vi "Check Path Length.vi"(8 "y":i32) -> (2 "Array":cluster{string, i32}[](array[cluster])=[{"", 141}, {"", 140}, {"", 145}, {"", 139}, {"", 129}, {"", 148}, {"", 114}, {"", 129}, {"", 127}, {"", 158}, {"", 146}, {"", 158}, {"", 147}, {"", 146}, {"", 152}, {"", 148}, {"", 155}, {"", 135}, {"", 149}, {"", 136}, {"", 152}, {"", 149}, {"", 154}, {"", 162}, {"", 163}, {"", 147}, {"", 177}, {"", 166}, {"", 149}, {"", 134}, {"", 134}, {"", 157}, {"", 167}, {"", 153}, {"", 153}, {"", 140}, {"", 159}, {"", 160}, {"", 163}, {"", 168}, {"", 167}, {"", 147}, {"", 161}, {"", 135}, {"", 147}, {"", 160}, {"", 161}, {"", 149}, {"", 156}, {"", 132}, {"", 128}, {"", 151}, {"", 154}, {"", 156}, {"", 160}, {"", 148}, {"", 143}, {"", 147}, {"", 143}, {"", 141}, {"", 143}, {"", 140}, {"", 170}, {"", 147}, {"", 147}, {"", 135}, {"", 134}, {"", 129}, {"", 179}, {"", 180}, {"", 166}, {"", 161}, {"", 175}, {"", 178}, {"", 186}, {"", 160}, {"", 160}, {"", 148}, {"", 152}, {"", 146}, {"", 152}, {"", 150}, {"", 150}, {"", 151}, {"", 151}, {"", 151}, {"", 141}, {"", 166}, {"", 154}, {"", 154}, {"", 155}, {"", 156}, {"", 167}, {"", 155}, {"", 171}, {"", 169}, {"", 158}, {"", 143}, {"", 160}, {"", 141}, {"", 156}, {"", 143}, {"", 151}, {"", 158}, {"", 159}, {"", 147}, {"", 154}, {"", 152}, {"", 150}, {"", 153}, {"", 161}, {"", 151}, {"", 144}, {"", 149}, {"", 145}, {"", 144}, {"", 150}, {"", 158}, {"", 159}, {"", 157}, {"", 154}, {"", 150}, {"", 154}, {"", 142}, {"", 152}, {"", 146}, {"", 152}, {"", 151}, {"", 144}, {"", 148}, {"", 136}, {"", 150}, {"", 154}, {"", 149}, {"", 129}, {"", 162}, {"", 163}, {"", 164}, {"", 160}, {"", 163}, {"", 152}, {"", 162}, {"", 172}, {"", 149}, {"", 151}, {"", 162}, {"", 153}, {"", 163}, {"", 162}, {"", 158}, {"", 170}, {"", 165}, {"", 163}, {"", 163}, {"", 173}, {"", 155}, {"", 174}, {"", 173}, {"", 169}, {"", 166}, {"", 159}, {"", 160}, {"", 153}, {"", 143}, {"", 144}, {"", 138}, {"", 139}, {"", 136}, {"", 147}, {"", 148}, {"", 144}, {"", 151}, {"", 154}, {"", 131}, {"", 128}, {"", 170}, {"", 146}, {"", 140}, {"", 157}, {"", 151}, {"", 152}, {"", 152}, {"", 151}, {"", 162}, {"", 145}, {"", 144}, {"", 145}, {"", 150}, {"", 162}, {"", 170}, {"", 135}, {"", 131}, {"", 131}, {"", 159}, {"", 142}, {"", 157}, {"", 157}, {"", 147}, {"", 149}, {"", 160}, {"", 145}, {"", 150}, {"", 147}, {"", 164}, {"", 153}, {"", 175}, {"", 158}, {"", 146}, {"", 142}, {"", 144}, {"", 154}, {"", 151}, {"", 151}, {"", 152}, {"", 147}, {"", 144}, {"", 146}, {"", 146}, {"", 152}, {"", 143}, {"", 146}, {"", 142}, {"", 158}, {"", 149}, {"", 144}, {"", 151}, {"", 137}, {"", 152}, {"", 160}, {"", 142}, {"", 164}, {"", 145}, {"", 141}, {"", 144}, {"", 138}, {"", 139}, {"", 149}, {"", 161}, {"", 138}, {"", 166}, {"", 132}, {"", 140}, {"", 136}, {"", 139}, {"", 140}, {"", 132}, {"", 137}, {"", 146}, {"", 143}, {"", 144}, {"", 148}, {"", 141}, {"", 149}, {"", 150}, {"", 179}, {"", 162}, {"", 175}, {"", 168}, {"", 169}, {"", 155}, {"", 150}, {"", 149}, {"", 155}, {"", 152}, {"", 180}, {"", 163}, {"", 163}, {"", 160}, {"", 160}, {"", 157}, {"", 158}, {"", 163}, {"", 165}, {"", 157}, {"", 165}, {"", 161}, {"", 155}, {"", 159}, {"", 160}, {"", 147}, {"", 166}, {"", 151}, {"", 150}, {"", 162}, {"", 158}, {"", 171}, {"", 155}, {"", 167}, {"", 169}, {"", 167}, {"", 171}, {"", 167}, {"", 171}, {"", 169}, {"", 173}, {"", 175}, {"", 162}, {"", 174}, {"", 172}, {"", 176}, {"", 173}, {"", 177}, {"", 175}, {"", 179}, {"", 175}, {"", 163}, {"", 149}, {"", 160}, {"", 151}, {"", 153}, {"", 149}, {"", 149}, {"", 150}, {"", 146}, {"", 155}, {"", 153}, {"", 156}, {"", 142}, {"", 141}, {"", 143}, {"", 143}, {"", 147}, {"", 141}, {"", 149}, {"", 149}, {"", 153}, {"", 157}, {"", 164}, {"", 162}, {"", 162}, {"", 146}, {"", 151}, {"", 153}, {"", 137}, {"", 141}, {"", 145}, {"", 156}, {"", 151}, {"", 147}, {"", 146}, {"", 145}, {"", 149}, {"", 145}, {"", 142}, {"", 145}, {"", 149}, {"", 150}, {"", 144}, {"", 148}, {"", 160}, {"", 148}, {"", 176}, {"", 144}, {"", 146}, {"", 153}, {"", 136}, {"", 136}, {"", 147}, {"", 163}, {"", 175}, {"", 178}, {"", 189}, {"", 177}, {"", 144}, {"", 157}, {"", 160}, {"", 171}, {"", 159}, {"", 179}, {"", 170}, {"", 176}, {"", 121}, {"", 178}, {"", 178}, {"", 179}, {"", 181}, {"", 182}, {"", 178}, {"", 177}, {"", 156}, {"", 183}, {"", 183}, {"", 181}, {"", 175}, {"", 165}, {"", 182}, {"", 191}, {"", 185}, {"", 158}, {"", 150}, {"", 181}, {"", 154}, {"", 177}, {"", 170}, {"", 208}, {"", 179}, {"", 191}, {"", 200}, {"", 183}, {"", 186}, {"", 198}, {"", 170}, {"", 183}, {"", 181}, {"", 181}, {"", 183}, {"", 198}, {"", 186}, {"", 176}, {"", 174}, {"", 181}, {"", 180}, {"", 182}, {"", 181}, {"", 196}, {"", 194}, {"", 192}, {"", 189}, {"", 195}, {"", 183}, {"", 147}, {"", 146}, {"", 142}, {"", 141}, {"", 128}, {"", 173}, {"", 168}, {"", 170}, {"", 154}, {"", 149}, {"", 171}, {"", 161}, {"", 158}, {"", 184}, {"", 162}, {"", 134}, {"", 178}, {"", 171}, {"", 185}, {"", 171}, {"", 167}, {"", 167}, {"", 169}, {"", 140}, {"", 169}, {"", 157}, {"", 168}, {"", 182}, {"", 186}, {"", 184}, {"", 148}, {"", 173}, {"", 141}, {"", 130}, {"", 154}, {"", 138}, {"", 131}, {"", 140}, {"", 132}, {"", 160}, {"", 150}, {"", 150}, {"", 154}, {"", 149}, {"", 175}, {"", 150}, {"", 152}, {"", 149}, {"", 152}, {"", 147}, {"", 149}, {"", 151}, {"", 154}, {"", 160}, {"", 144}, {"", 166}, {"", 148}, {"", 155}, {"", 151}, {"", 155}, {"", 151}, {"", 143}, {"", 159}, {"", 135}, {"", 159}, {"", 175}, {"", 139}, {"", 159}, {"", 160}, {"", 153}, {"", 147}, {"", 148}, {"", 140}, {"", 144}, {"", 140}, {"", 147}, {"", 146}, {"", 139}, {"", 149}, {"", 163}, {"", 162}, {"", 165}, {"", 165}, {"", 154}, {"", 155}, {"", 137}, {"", 158}, {"", 147}, {"", 146}, {"", 151}, {"", 148}, {"", 158}, {"", 159}, {"", 155}, {"", 154}, {"", 125}, {"", 138}, {"", 131}, {"", 144}, {"", 139}, {"", 133}, {"", 140}, {"", 137}, {"", 145}, {"", 131}, {"", 146}, {"", 138}, {"", 122}, {"", 143}, {"", 138}, {"", 140}, {"", 146}, {"", 147}, {"", 140}, {"", 136}, {"", 140}, {"", 139}, {"", 134}, {"", 138}, {"", 122}, {"", 147}, {"", 155}, {"", 159}, {"", 142}, {"", 147}, {"", 145}, {"", 140}, {"", 150}, {"", 142}, {"", 150}, {"", 147}, {"", 167}, {"", 163}, {"", 165}], 3 "Waveform Graph":i32[](graph)=[141, 140, 145, 139, 129, 148, 114, 129, 127, 158, 146, 158, 147, 146, 152, 148, 155, 135, 149, 136, 152, 149, 154, 162, 163, 147, 177, 166, 149, 134, 134, 157, 167, 153, 153, 140, 159, 160, 163, 168, 167, 147, 161, 135, 147, 160, 161, 149, 156, 132, 128, 151, 154, 156, 160, 148, 143, 147, 143, 141, 143, 140, 170, 147, 147, 135, 134, 129, 179, 180, 166, 161, 175, 178, 186, 160, 160, 148, 152, 146, 152, 150, 150, 151, 151, 151, 141, 166, 154, 154, 155, 156, 167, 155, 171, 169, 158, 143, 160, 141, 156, 143, 151, 158, 159, 147, 154, 152, 150, 153, 161, 151, 144, 149, 145, 144, 150, 158, 159, 157, 154, 150, 154, 142, 152, 146, 152, 151, 144, 148, 136, 150, 154, 149, 129, 162, 163, 164, 160, 163, 152, 162, 172, 149, 151, 162, 153, 163, 162, 158, 170, 165, 163, 163, 173, 155, 174, 173, 169, 166, 159, 160, 153, 143, 144, 138, 139, 136, 147, 148, 144, 151, 154, 131, 128, 170, 146, 140, 157, 151, 152, 152, 151, 162, 145, 144, 145, 150, 162, 170, 135, 131, 131, 159, 142, 157, 157, 147, 149, 160, 145, 150, 147, 164, 153, 175, 158, 146, 142, 144, 154, 151, 151, 152, 147, 144, 146, 146, 152, 143, 146, 142, 158, 149, 144, 151, 137, 152, 160, 142, 164, 145, 141, 144, 138, 139, 149, 161, 138, 166, 132, 140, 136, 139, 140, 132, 137, 146, 143, 144, 148, 141, 149, 150, 179, 162, 175, 168, 169, 155, 150, 149, 155, 152, 180, 163, 163, 160, 160, 157, 158, 163, 165, 157, 165, 161, 155, 159, 160, 147, 166, 151, 150, 162, 158, 171, 155, 167, 169, 167, 171, 167, 171, 169, 173, 175, 162, 174, 172, 176, 173, 177, 175, 179, 175, 163, 149, 160, 151, 153, 149, 149, 150, 146, 155, 153, 156, 142, 141, 143, 143, 147, 141, 149, 149, 153, 157, 164, 162, 162, 146, 151, 153, 137, 141, 145, 156, 151, 147, 146, 145, 149, 145, 142, 145, 149, 150, 144, 148, 160, 148, 176, 144, 146, 153, 136, 136, 147, 163, 175, 178, 189, 177, 144, 157, 160, 171, 159, 179, 170, 176, 121, 178, 178, 179, 181, 182, 178, 177, 156, 183, 183, 181, 175, 165, 182, 191, 185, 158, 150, 181, 154, 177, 170, 208, 179, 191, 200, 183, 186, 198, 170, 183, 181, 181, 183, 198, 186, 176, 174, 181, 180, 182, 181, 196, 194, 192, 189, 195, 183, 147, 146, 142, 141, 128, 173, 168, 170, 154, 149, 171, 161, 158, 184, 162, 134, 178, 171, 185, 171, 167, 167, 169, 140, 169, 157, 168, 182, 186, 184, 148, 173, 141, 130, 154, 138, 131, 140, 132, 160, 150, 150, 154, 149, 175, 150, 152, 149, 152, 147, 149, 151, 154, 160, 144, 166, 148, 155, 151, 155, 151, 143, 159, 135, 159, 175, 139, 159, 160, 153, 147, 148, 140, 144, 140, 147, 146, 139, 149, 163, 162, 165, 165, 154, 155, 137, 158, 147, 146, 151, 148, 158, 159, 155, 154, 125, 138, 131, 144, 139, 133, 140, 137, 145, 131, 146, 138, 122, 143, 138, 140, 146, 147, 140, 136, 140, 139, 134, 138, 122, 147, 155, 159, 142, 147, 145, 140, 150, 142, 150, 147, 167, 163, 165])   [LabVIEW 2017, in "testcase-documentation.lvclass"]
uses:
  testcase-documentation.lvclass
  src/user.lib/_NEVSTOP/Communicable State Machine(CSM)/_Shared/CSM Shared.lvlib
panel:
  out "All Files in Dir":path[](array[path])=[path "C:/Program Files (x86)/National Instruments/LabVIEW 2017/user.lib/_NEVSTOP/Communicable State Machine(CSM)/Add State(s) to Queue By BOOL++.vi", path "C:/Program Files (x86)/National Instruments/LabVIEW 2017/user.lib/_NEVSTOP/Communicable State Machine(CSM)/Build Message with Arguments++.vi", path "C:/Program Files (x86)/National Instruments/LabVIEW 2017/user.lib/_NEVSTOP/Communicable State Machine(CSM)/Build State String with Arguments++.vi", path "C:/Program Files (x86)/National Instruments/LabVIEW 2017/user.lib/_NEVSTOP/Communicable State Machine(CSM)/Communicable State Machine.lvlib", path "C:/Program Files (x86)/National Instruments/LabVIEW 2017/user.lib/_NEVSTOP/Communicable State Machine(CSM)/CSM Module Template.vi", path "C:/Program Files (x86)/National Instruments/LabVIEW 2017/user.lib/_NEVSTOP/Communicable State Machine(CSM)/CSM User Interface(UI) Module Template.vi", path "C:/Program Files (x86)/National Instruments/LabVIEW 2017/user.lib/_NEVSTOP/Communicable State Machine(CSM)/dir.mnu", path "C:/Program Files (x86)/National Instruments/LabVIEW 2017/user.lib/_NEVSTOP/Communicable State Machine(CSM)/Parse State Queue++.vi", path "C:/Program Files (x86)/National Instruments/LabVIEW 2017/user.lib/_NEVSTOP/Communicable State Machine(CSM)/_csmDoc/csmdoc.lvlib", path "C:/Program Files (x86)/National Instruments/LabVIEW 2017/user.lib/_NEVSTOP/Communicable State Machine(CSM)/_csmDoc/csmdoc_export_all_csm_VI_description_doc.vi", path "C:/Program Files (x86)/National Instruments/LabVIEW 2017/user.lib/_NEVSTOP/Communicable State Machine(CSM)/_csmDoc/csmdoc_export_VI_description.vi", path "C:/Program Files (x86)/National Instruments/LabVIEW 2017/user.lib/_NEVSTOP/Communicable State Machine(CSM)/_csmDoc/csmdoc_import_all_csm_VI_description_doc.vi", path "C:/Program Files (x86)/National Instruments/LabVIEW 2017/user.lib/_NEVSTOP/Communicable State Machine(CSM)/_csmDoc/csmdoc_import_doc_to_singleVI.vi", path "C:/Program Files (x86)/National Instruments/LabVIEW 2017/user.lib/_NEVSTOP/Communicable State Machine(CSM)/_csmDoc/csmdoc_import_VI_description.vi", path "C:/Program Files (x86)/National Instruments/LabVIEW 2017/user.lib/_NEVSTOP/Communicable State Machine(CSM)/_csmDoc/csmdoc_list_all_csm_documented_VIs.vi", path "C:/Program Files (x86)/National Instruments/LabVIEW 2017/user.lib/_NEVSTOP/Communicable State Machine(CSM)/_csmDoc/csmdoc_load vi description map.vi", path "C:/Program Files (x86)/National Instruments/LabVIEW 2017/user.lib/_NEVSTOP/Communicable State Machine(CSM)/_csmDoc/Support/Parse VI Documentation String.vi", path "C:/Program Files (x86)/National Instruments/LabVIEW 2017/user.lib/_NEVSTOP/Communicable State Machine(CSM)/_csmHelper/CSM-Helper API.vi", path "C:/Program Files (x86)/National Instruments/LabVIEW 2017/user.lib/_NEVSTOP/Communicable State Machine(CSM)/_csmHelper/CSM-Helper usecase Template.vit", path "C:/Program Files (x86)/National Instruments/LabVIEW 2017/user.lib/_NEVSTOP/Communicable State Machine(CSM)/_csmHelper/CSM-Helper.lvclass", path "C:/Program Files (x86)/National Instruments/LabVIEW 2017/user.lib/_NEVSTOP/Communicable State Machine(CSM)/_csmHelper/_support/_Add VI Reference Case.vi", path "C:/Program Files (x86)/National Instruments/LabVIEW 2017/user.lib/_NEVSTOP/Communicable State Machine(CSM)/_csmHelper/_support/Connect Information.vi", path "C:/Program Files (x86)/National Instruments/LabVIEW 2017/user.lib/_NEVSTOP/Communicable State Machine(CSM)/_csmHelper/_support/Diagram Node Information.vi", path "C:/Program Files (x86)/National Instruments/LabVIEW 2017/user.lib/_NEVSTOP/Communicable State Machine(CSM)/_csmHelper/_support/Get Argument Info From back Term.vi", path "C:/Program Files (x86)/National Instruments/LabVIEW 2017/user.lib/_NEVSTOP/Communicable State Machine(CSM)/_csmHelper/_support/Get Argument Info From Front Term.vi", path "C:/Program Files (x86)/National Instruments/LabVIEW 2017/user.lib/_NEVSTOP/Communicable State Machine(CSM)/_csmHelper/_support/GObject Terminals.vi", path "C:/Program Files (x86)/National Instruments/LabVIEW 2017/user.lib/_NEVSTOP/Communicable State Machine(CSM)/_csmHelper/_support/Relative Pos to InterData Tunnel of CaseContent.vi", path "C:/Program Files (x86)/National Instruments/LabVIEW 2017/user.lib/_NEVSTOP/Communicable State Machine(CSM)/_csmHelper/_support/Resize CaseStructure By Making Space.vi", path "C:/Program Files (x86)/National Instruments/LabVIEW 2017/user.lib/_NEVSTOP/Communicable State Machine(CSM)/_csmHelper/_support/Search With Pattern.vi", path "C:/Program Files (x86)/National Instruments/LabVIEW 2017/user.lib/_NEVSTOP/Communicable State Machine(CSM)/_csmHelper/_support/sub1.vi", path "C:/Program Files (x86)/National Instruments/LabVIEW 2017/user.lib/_NEVSTOP/Communicable State Machine(CSM)/_csmHelper/_support/sub2.vi", path "C:/Program Files (x86)/National Instruments/LabVIEW 2017/user.lib/_NEVSTOP/Communicable State Machine(CSM)/_csmHelper/_support/Creation/Refresh References.vi", path "C:/Program Files (x86)/National Instruments/LabVIEW 2017/user.lib/_NEVSTOP/Communicable State Machine(CSM)/_csmHelper/_support/Refs/Get ParentRef Until Type Matched.vi", path "C:/Program Files (x86)/National Instruments/LabVIEW 2017/user.lib/_NEVSTOP/Communicable State Machine(CSM)/_csmHelper/_support/Refs/Is in JKISM or CSM.vi", path "C:/Program Files (x86)/National Instruments/LabVIEW 2017/user.lib/_NEVSTOP/Communicable State Machine(CSM)/_csmHelper/_support/Refs/Relationship Check.vi", path "C:/Program Files (x86)/National Instruments/LabVIEW 2017/user.lib/_NEVSTOP/Communicable State Machine(CSM)/_csmHelper/API/Add State Frame.vi", path "C:/Program Files (x86)/National Instruments/LabVIEW 2017/user.lib/_NEVSTOP/Communicable State Machine(CSM)/_csmHelper/API/Check NewStateNotify is Registered.vi", path "C:/Program Files (x86)/National Instruments/LabVIEW 2017/user.lib/_NEVSTOP/Communicable State Machine(CSM)/_csmHelper/API/Connect Error Wire If not Connected.vi", path "C:/Program Files (x86)/National Instruments/LabVIEW 2017/user.lib/_NEVSTOP/Communicable State Machine(CSM)/_csmHelper/API/Connect EventReg Wire If not Connected.vi", path "C:/Program Files (x86)/National Instruments/LabVIEW 2017/user.lib/_NEVSTOP/Communicable State Machine(CSM)/_csmHelper/API/Connect Internal Data Wire If not Connected.vi", path "C:/Program Files (x86)/National Instruments/LabVIEW 2017/user.lib/_NEVSTOP/Communicable State Machine(CSM)/_csmHelper/API/Connect LastResp to Response in Error Case.vi", path "C:/Program Files (x86)/National Instruments/LabVIEW 2017/user.lib/_NEVSTOP/Communicable State Machine(CSM)/_csmHelper/API/Connect Paired Tunnels.vi", path "C:/Program Files (x86)/National Instruments/LabVIEW 2017/user.lib/_NEVSTOP/Communicable State Machine(CSM)/_csmHelper/API/Connect StateQ Wire If not Connected.vi", path "C:/Program Files (x86)/National Instruments/LabVIEW 2017/user.lib/_NEVSTOP/Communicable State Machine(CSM)/_csmHelper/API/Copy State.vi", path "C:/Program Files (x86)/National Instruments/LabVIEW 2017/user.lib/_NEVSTOP/Communicable State Machine(CSM)/_csmHelper/API/Create From Basic Refs.vi", path "C:/Program Files (x86)/National Instruments/LabVIEW 2017/user.lib/_NEVSTOP/Communicable State Machine(CSM)/_csmHelper/API/Create From CaseStructure Reference.vi", path "C:/Program Files (x86)/National Instruments/LabVIEW 2017/user.lib/_NEVSTOP/Communicable State Machine(CSM)/_csmHelper/API/Create From EventStructure Reference.vi", path "C:/Program Files (x86)/National Instruments/LabVIEW 2017/user.lib/_NEVSTOP/Communicable State Machine(CSM)/_csmHelper/API/Create From VI Reference.vi", path "C:/Program Files (x86)/National Instruments/LabVIEW 2017/user.lib/_NEVSTOP/Communicable State Machine(CSM)/_csmHelper/API/Create From WhileLoop Reference.vi", path "C:/Program Files (x86)/National Instruments/LabVIEW 2017/user.lib/_NEVSTOP/Communicable State Machine(CSM)/_csmHelper/API/Destroy.vi", path "C:/Program Files (x86)/National Instruments/LabVIEW 2017/user.lib/_NEVSTOP/Communicable State Machine(CSM)/_csmHelper/API/Doc.vi", path "C:/Program Files (x86)/National Instruments/LabVIEW 2017/user.lib/_NEVSTOP/Communicable State Machine(CSM)/_csmHelper/API/Get All API Interface Info.vi", path "C:/Program Files (x86)/National Instruments/LabVIEW 2017/user.lib/_NEVSTOP/Communicable State Machine(CSM)/_csmHelper/API/Get All Status Interface Info.vi", path "C:/Program Files (x86)/National Instruments/LabVIEW 2017/user.lib/_NEVSTOP/Communicable State Machine(CSM)/_csmHelper/API/Get CaseFrame Index By CaseName.vi", path "C:/Program Files (x86)/National Instruments/LabVIEW 2017/user.lib/_NEVSTOP/Communicable State Machine(CSM)/_csmHelper/API/Get CaseFrame Reference By CaseName.vi", path "C:/Program Files (x86)/National Instruments/LabVIEW 2017/user.lib/_NEVSTOP/Communicable State Machine(CSM)/_csmHelper/API/Get Event Structure Num.vi", path "C:/Program Files (x86)/National Instruments/LabVIEW 2017/user.lib/_NEVSTOP/Communicable State Machine(CSM)/_csmHelper/API/Get Interface Info.vi", path "C:/Program Files (x86)/National Instruments/LabVIEW 2017/user.lib/_NEVSTOP/Communicable State Machine(CSM)/_csmHelper/API/Get Internal Data Info.vi", path "C:/Program Files (x86)/National Instruments/LabVIEW 2017/user.lib/_NEVSTOP/Communicable State Machine(CSM)/_csmHelper/API/Open Block Diagram.vi", path "C:/Program Files (x86)/National Instruments/LabVIEW 2017/user.lib/_NEVSTOP/Communicable State Machine(CSM)/_csmHelper/API/Open Front Panel.vi", path "C:/Program Files (x86)/National Instruments/LabVIEW 2017/user.lib/_NEVSTOP/Communicable State Machine(CSM)/_csmHelper/API/Remove State Frame.vi", path "C:/Program Files (x86)/National Instruments/LabVIEW 2017/user.lib/_NEVSTOP/Communicable State Machine(CSM)/_csmHelper/API/Save Instrument.vi", path "C:/Program Files (x86)/National Instruments/LabVIEW 2017/user.lib/_NEVSTOP/Communicable State Machine(CSM)/_csmHelper/API/Set Error Tunnel Use Default If not Connected.vi", path "C:/Program Files (x86)/National Instruments/LabVIEW 2017/user.lib/_NEVSTOP/Communicable State Machine(CSM)/_csmHelper/API/Set Visible Case Frame.vi", path "C:/Program Files (x86)/National Instruments/LabVIEW 2017/user.lib/_NEVSTOP/Communicable State Machine(CSM)/_csmHelper/API/Set Wire Label Visible.vi", path "C:/Program Files (x86)/National Instruments/LabVIEW 2017/user.lib/_NEVSTOP/Communicable State Machine(CSM)/_csmHelper/API/Start Undo.vi", path "C:/Program Files (x86)/National Instruments/LabVIEW 2017/user.lib/_NEVSTOP/Communicable State Machine(CSM)/_csmHelper/API/Stop Undo.vi", path "C:/Program Files (x86)/National Instruments/LabVIEW 2017/user.lib/_NEVSTOP/Communicable State Machine(CSM)/_csmHelper/API/Undo.vi", path "C:/Program Files (x86)/National Instruments/LabVIEW 2017/user.lib/_NEVSTOP/Communicable State Machine(CSM)/_csmHelper/API with lvcsm Support/_Read StringList with lvcsm Support.vi", path "C:/Program Files (x86)/National Instruments/LabVIEW 2017/user.lib/_NEVSTOP/Communicable State Machine(CSM)/_csmHelper/API with lvcsm Support/CSM-Helper API with lvcsm Support.lvlib", path "C:/Program Files (x86)/National Instruments/LabVIEW 2017/user.lib/_NEVSTOP/Communicable State Machine(CSM)/_csmHelper/API with lvcsm Support/CSM-Helper API(lvcsm).mnu", path "C:/Program Files (x86)/National Instruments/LabVIEW 2017/user.lib/_NEVSTOP/Communicable State Machine(CSM)/_csmHelper/API with lvcsm Support/Jump to CSM State.vi", path "C:/Program Files (x86)/National Instruments/LabVIEW 2017/user.lib/_NEVSTOP/Communicable State Machine(CSM)/_csmHelper/API with lvcsm Support/Read CSM API with lvcsm Support.vi", path "C:/Program Files (x86)/National Instruments/LabVIEW 2017/user.lib/_NEVSTOP/Communicable State Machine(CSM)/_csmHelper/API with lvcsm Support/Read CSM States with lvcsm Support.vi", path "C:/Program Files (x86)/National Instruments/LabVIEW 2017/user.lib/_NEVSTOP/Communicable State Machine(CSM)/_csmHelper/API with lvcsm Support/Read CSM UserDef States with lvcsm Support.vi", path "C:/Program Files (x86)/National Instruments/LabVIEW 2017/user.lib/_NEVSTOP/Communicable State Machine(CSM)/_csmHelper/lvcsmFile/_Common Path to Specific Path.vi", path "C:/Program Files (x86)/National Instruments/LabVIEW 2017/user.lib/_NEVSTOP/Communicable State Machine(CSM)/_csmHelper/lvcsmFile/_Specific Path to Common Path.vi", path "C:/Program Files (x86)/National Instruments/LabVIEW 2017/user.lib/_NEVSTOP/Communicable State Machine(CSM)/_csmHelper/lvcsmFile/_System Locations.vi", path "C:/Program Files (x86)/National Instruments/LabVIEW 2017/user.lib/_NEVSTOP/Communicable State Machine(CSM)/_csmHelper/lvcsmFile/Change File Extension.vi", path "C:/Program Files (x86)/National Instruments/LabVIEW 2017/user.lib/_NEVSTOP/Communicable State Machine(CSM)/_csmHelper/lvcsmFile/lvcsm File Path.vi", path "C:/Program Files (x86)/National Instruments/LabVIEW 2017/user.lib/_NEVSTOP/Communicable State Machine(CSM)/_csmHelper/lvcsmFile/lvcsm File Support.lvlib", path "C:/Program Files (x86)/National Instruments/LabVIEW 2017/user.lib/_NEVSTOP/Communicable State Machine(CSM)/_csmHelper/lvcsmFile/lvcsm File Support.mnu", path "C:/Program Files (x86)/National Instruments/LabVIEW 2017/user.lib/_NEVSTOP/Communicable State Machine(CSM)/_csmHelper/lvcsmFile/lvcsm Read Cluster.vim", path "C:/Program Files (x86)/National Instruments/LabVIEW 2017/user.lib/_NEVSTOP/Communicable State Machine(CSM)/_csmHelper/lvcsmFile/lvcsm String to Path.vi", path "C:/Program Files (x86)/National Instruments/LabVIEW 2017/user.lib/_NEVSTOP/Communicable State Machine(CSM)/_csmHelper/lvcsmFile/lvcsm Write Cluster.vim", path "C:/Program Files (x86)/National Instruments/LabVIEW 2017/user.lib/_NEVSTOP/Communicable State Machine(CSM)/_csmHelper/lvcsmFile/Path to lvcsm String.vi", path "C:/Program Files (x86)/National Instruments/LabVIEW 2017/user.lib/_NEVSTOP/Communicable State Machine(CSM)/_csmHelper/Properties/Read APIs.vi", path "C:/Program Files (x86)/National Instruments/LabVIEW 2017/user.lib/_NEVSTOP/Communicable State Machine(CSM)/_csmHelper/Properties/Read Back Tunnel Internal TermRefs.vi", path "C:/Program Files (x86)/National Instruments/LabVIEW 2017/user.lib/_NEVSTOP/Communicable State Machine(CSM)/_csmHelper/Properties/Read Back Tunnels Refs.vi", path "C:/Program Files (x86)/National Instruments/LabVIEW 2017/user.lib/_NEVSTOP/Communicable State Machine(CSM)/_csmHelper/Properties/Read Block Diagram Ref.vi", path "C:/Program Files (x86)/National Instruments/LabVIEW 2017/user.lib/_NEVSTOP/Communicable State Machine(CSM)/_csmHelper/Properties/Read Case Structure Ref.vi", path "C:/Program Files (x86)/National Instruments/LabVIEW 2017/user.lib/_NEVSTOP/Communicable State Machine(CSM)/_csmHelper/Properties/Read Event Structure Ref.vi", path "C:/Program Files (x86)/National Instruments/LabVIEW 2017/user.lib/_NEVSTOP/Communicable State Machine(CSM)/_csmHelper/Properties/Read Front Tunnel Internal TermRefs.vi", path "C:/Program Files (x86)/National Instruments/LabVIEW 2017/user.lib/_NEVSTOP/Communicable State Machine(CSM)/_csmHelper/Properties/Read Front Tunnels Refs.vi", path "C:/Program Files (x86)/National Instruments/LabVIEW 2017/user.lib/_NEVSTOP/Communicable State Machine(CSM)/_csmHelper/Properties/Read New State Notifier Event State Ref.vi", path "C:/Program Files (x86)/National Instruments/LabVIEW 2017/user.lib/_NEVSTOP/Communicable State Machine(CSM)/_csmHelper/Properties/Read Paired Tunnels of Case Structure.vi", path "C:/Program Files (x86)/National Instruments/LabVIEW 2017/user.lib/_NEVSTOP/Communicable State Machine(CSM)/_csmHelper/Properties/Read Parse State Queue Ref.vi", path "C:/Program Files (x86)/National Instruments/LabVIEW 2017/user.lib/_NEVSTOP/Communicable State Machine(CSM)/_csmHelper/Properties/Read States.vi", path "C:/Program Files (x86)/National Instruments/LabVIEW 2017/user.lib/_NEVSTOP/Communicable State Machine(CSM)/_csmHelper/Properties/Read Timeout Event State Ref.vi", path "C:/Program Files (x86)/National Instruments/LabVIEW 2017/user.lib/_NEVSTOP/Communicable State Machine(CSM)/_csmHelper/Properties/Read Type.vi", path "C:/Program Files (x86)/National Instruments/LabVIEW 2017/user.lib/_NEVSTOP/Communicable State Machine(CSM)/_csmHelper/Properties/Read User-Defined States.vi", path "C:/Program Files (x86)/National Instruments/LabVIEW 2017/user.lib/_NEVSTOP/Communicable State Machine(CSM)/_csmHelper/Properties/Read VI Ref.vi", path "C:/Program Files (x86)/National Instruments/LabVIEW 2017/user.lib/_NEVSTOP/Communicable State Machine(CSM)/_csmHelper/Properties/Read While Loop Ref.vi", path "C:/Program Files (x86)/National Instruments/LabVIEW 2017/user.lib/_NEVSTOP/Communicable State Machine(CSM)/_csmHelper/Typedef/_csmhelper_Back_Tunnels_Refs.ctl", path "C:/Program Files (x86)/National Instruments/LabVIEW 2017/user.lib/_NEVSTOP/Communicable State Machine(CSM)/_csmHelper/Typedef/_csmhelper_Front_Tunnels_Refs.ctl", path "C:/Program Files (x86)/National Instruments/LabVIEW 2017/user.lib/_NEVSTOP/Communicable State Machine(CSM)/_csmHelper/Typedef/Def-Argument Info.ctl", path "C:/Program Files (x86)/National Instruments/LabVIEW 2017/user.lib/_NEVSTOP/Communicable State Machine(CSM)/_csmHelper/Typedef/Def-Conncted Information.ctl", path "C:/Program Files (x86)/National Instruments/LabVIEW 2017/user.lib/_NEVSTOP/Communicable State Machine(CSM)/_csmHelper/Typedef/Def-Internal Data Info.ctl", path "C:/Program Files (x86)/National Instruments/LabVIEW 2017/user.lib/_NEVSTOP/Communicable State Machine(CSM)/_csmHelper/usecase/Add VI Reference Case.vi", path "C:/Program Files (x86)/National Instruments/LabVIEW 2017/user.lib/_NEVSTOP/Communicable State Machine(CSM)/_csmHelper/usecase/Remove All CSM Bookmarks.vi", path "C:/Program Files (x86)/National Instruments/LabVIEW 2017/user.lib/_NEVSTOP/Communicable State Machine(CSM)/_csmHelper/usecase/Replace Debug Log History Method.vi", path "C:/Program Files (x86)/National Instruments/LabVIEW 2017/user.lib/_NEVSTOP/Communicable State Machine(CSM)/_csmHelper/usecase/standardize CSM Module.vi", path "C:/Program Files (x86)/National Instruments/LabVIEW 2017/user.lib/_NEVSTOP/Communicable State Machine(CSM)/_csmHelper/Utility/CSM Basic Refs.ctl", path "C:/Program Files (x86)/National Instruments/LabVIEW 2017/user.lib/_NEVSTOP/Communicable State Machine(CSM)/_csmHelper/Utility/CSM Essential States.vi", path "C:/Program Files (x86)/National Instruments/LabVIEW 2017/user.lib/_NEVSTOP/Communicable State Machine(CSM)/_csmHelper/Utility/CSM Module Type.ctl", path "C:/Program Files (x86)/National Instruments/LabVIEW 2017/user.lib/_NEVSTOP/Communicable State Machine(CSM)/_csmHelper/Utility/CSM Module Type.vi", path "C:/Program Files (x86)/National Instruments/LabVIEW 2017/user.lib/_NEVSTOP/Communicable State Machine(CSM)/_csmHelper/Utility/CSM-Helper Utility.lvlib", path "C:/Program Files (x86)/National Instruments/LabVIEW 2017/user.lib/_NEVSTOP/Communicable State Machine(CSM)/_csmHelper/Utility/Is CSM Module - CaseStructure.vi", path "C:/Program Files (x86)/National Instruments/LabVIEW 2017/user.lib/_NEVSTOP/Communicable State Machine(CSM)/_csmHelper/Utility/Is CSM Module - EventStructure.vi", path "C:/Program Files (x86)/National Instruments/LabVIEW 2017/user.lib/_NEVSTOP/Communicable State Machine(CSM)/_csmHelper/Utility/Is CSM Module - ParseStateVI.vi", path "C:/Program Files (x86)/National Instruments/LabVIEW 2017/user.lib/_NEVSTOP/Communicable State Machine(CSM)/_csmHelper/Utility/Is CSM Module - Structure.vi", path "C:/Program Files (x86)/National Instruments/LabVIEW 2017/user.lib/_NEVSTOP/Communicable State Machine(CSM)/_csmHelper/Utility/Is CSM Module - VIRef.vi", path "C:/Program Files (x86)/National Instruments/LabVIEW 2017/user.lib/_NEVSTOP/Communicable State Machine(CSM)/_csmHelper/Utility/Is CSM Module - WhileLoop.vi", path "C:/Program Files (x86)/National Instruments/LabVIEW 2017/user.lib/_NEVSTOP/Communicable State Machine(CSM)/_csmHelper/Utility/Is CSM Module.vi", path "C:/Program Files (x86)/National Instruments/LabVIEW 2017/user.lib/_NEVSTOP/Communicable State Machine(CSM)/_csmHelper/Utility/_Support/CaseStructure.llb", path "C:/Program Files (x86)/National Instruments/LabVIEW 2017/user.lib/_NEVSTOP/Communicable State Machine(CSM)/_csmHelper/Utility/_Support/Diagram.llb", path "C:/Program Files (x86)/National Instruments/LabVIEW 2017/user.lib/_NEVSTOP/Communicable State Machine(CSM)/_csmHelper/Utility/_Support/PairedTunnels.llb", path "C:/Program Files (x86)/National Instruments/LabVIEW 2017/user.lib/_NEVSTOP/Communicable State Machine(CSM)/_csmHelper/Utility/_Support/Relationship.llb", path "C:/Program Files (x86)/National Instruments/LabVIEW 2017/user.lib/_NEVSTOP/Communicable State Machine(CSM)/_csmHelper/Utility/_Support/SubVI.llb", path "C:/Program Files (x86)/National Instruments/LabVIEW 2017/user.lib/_NEVSTOP/Communicable State Machine(CSM)/_csmHelper/Utility/_Support/Terminals.llb", path "C:/Program Files (x86)/National Instruments/LabVIEW 2017/user.lib/_NEVSTOP/Communicable State Machine(CSM)/_Documentation/_JKIHelper.mnu", path "C:/Program Files (x86)/National Instruments/LabVIEW 2017/user.lib/_NEVSTOP/Communicable State Machine(CSM)/_Documentation/CSM - Copyright QuickDrop.vi", path "C:/Program Files (x86)/National Instruments/LabVIEW 2017/user.lib/_NEVSTOP/Communicable State Machine(CSM)/_Documentation/CSM - Documentation QuickDrop.vi", path "C:/Program Files (x86)/National Instruments/LabVIEW 2017/user.lib/_NEVSTOP/Communicable State Machine(CSM)/_Documentation/CSM - Keywords QuickDrop.vi", path "C:/Program Files (x86)/National Instruments/LabVIEW 2017/user.lib/_NEVSTOP/Communicable State Machine(CSM)/_Documentation/dir.mnu", path "C:/Program Files (x86)/National Instruments/LabVIEW 2017/user.lib/_NEVSTOP/Communicable State Machine(CSM)/_Polymophic/Add State(s) to Queue By BOOL(Array All).vi", path "C:/Program Files (x86)/National Instruments/LabVIEW 2017/user.lib/_NEVSTOP/Communicable State Machine(CSM)/_Polymophic/Add State(s) to Queue By BOOL(Array Left).vi", path "C:/Program Files (x86)/National Instruments/LabVIEW 2017/user.lib/_NEVSTOP/Communicable State Machine(CSM)/_Polymophic/Add State(s) to Queue By BOOL(Array Right).vi", path "C:/Program Files (x86)/National Instruments/LabVIEW 2017/user.lib/_NEVSTOP/Communicable State Machine(CSM)/_Polymophic/Add State(s) to Queue By BOOL(Element).vi", path "C:/Program Files (x86)/National Instruments/LabVIEW 2017/user.lib/_NEVSTOP/Communicable State Machine(CSM)/_Polymophic/Build Asynchronous Message with Arguments.vi", path "C:/Program Files (x86)/National Instruments/LabVIEW 2017/user.lib/_NEVSTOP/Communicable State Machine(CSM)/_Polymophic/Build Interrupt Status Message.vi", path "C:/Program Files (x86)/National Instruments/LabVIEW 2017/user.lib/_NEVSTOP/Communicable State Machine(CSM)/_Polymophic/Build Message with Arguments(Auto Check).vi", path "C:/Program Files (x86)/National Instruments/LabVIEW 2017/user.lib/_NEVSTOP/Communicable State Machine(CSM)/_Polymophic/Build No-Reply Asynchronous Message with Arguments.vi", path "C:/Program Files (x86)/National Instruments/LabVIEW 2017/user.lib/_NEVSTOP/Communicable State Machine(CSM)/_Polymophic/Build Normal Status Message.vi", path "C:/Program Files (x86)/National Instruments/LabVIEW 2017/user.lib/_NEVSTOP/Communicable State Machine(CSM)/_Polymophic/Build Register Status Message.vi", path "C:/Program Files (x86)/National Instruments/LabVIEW 2017/user.lib/_NEVSTOP/Communicable State Machine(CSM)/_Polymophic/Build Synchronous Message with Arguments.vi", path "C:/Program Files (x86)/National Instruments/LabVIEW 2017/user.lib/_NEVSTOP/Communicable State Machine(CSM)/_Polymophic/Build Unregister Status Message.vi", path "C:/Program Files (x86)/National Instruments/LabVIEW 2017/user.lib/_NEVSTOP/Communicable State Machine(CSM)/_popupMenuPlugin/CSM Execute - Fix VI Reference State.vi", path "C:/Program Files (x86)/National Instruments/LabVIEW 2017/user.lib/_NEVSTOP/Communicable State Machine(CSM)/_popupMenuPlugin/CSM Execute - Highlight All Scripts.vi", path "C:/Program Files (x86)/National Instruments/LabVIEW 2017/user.lib/_NEVSTOP/Communicable State Machine(CSM)/_popupMenuPlugin/CSM Execute - Highlight Scripts.vi", path "C:/Program Files (x86)/National Instruments/LabVIEW 2017/user.lib/_NEVSTOP/Communicable State Machine(CSM)/_popupMenuPlugin/CSM Execute - Make String Safe as Arguments.vi", path "C:/Program Files (x86)/National Instruments/LabVIEW 2017/user.lib/_NEVSTOP/Communicable State Machine(CSM)/_popupMenuPlugin/CSM Execute - Remove all CSM Bookmarks.vi", path "C:/Program Files (x86)/National Instruments/LabVIEW 2017/user.lib/_NEVSTOP/Communicable State Machine(CSM)/_popupMenuPlugin/CSM Execute - Revert CSM Safe String.vi", path "C:/Program Files (x86)/National Instruments/LabVIEW 2017/user.lib/_NEVSTOP/Communicable State Machine(CSM)/_popupMenuPlugin/CSM Execute - Shortcut Menu Plug-In.ctl", path "C:/Program Files (x86)/National Instruments/LabVIEW 2017/user.lib/_NEVSTOP/Communicable State Machine(CSM)/_popupMenuPlugin/CSM Execute - Upgrade Debug Log History Method.vi", path "C:/Program Files (x86)/National Instruments/LabVIEW 2017/user.lib/_NEVSTOP/Communicable State Machine(CSM)/_popupMenuPlugin/_support/_CSM Scripts Colors.vi", path "C:/Program Files (x86)/National Instruments/LabVIEW 2017/user.lib/_NEVSTOP/Communicable State Machine(CSM)/_popupMenuPlugin/_support/_Highlight CSM Scripts(StringConstant).vi", path "C:/Program Files (x86)/National Instruments/LabVIEW 2017/user.lib/_NEVSTOP/Communicable State Machine(CSM)/_popupMenuPlugin/_support/_Highlight CSM Scripts(StringControl).vi", path "C:/Program Files (x86)/National Instruments/LabVIEW 2017/user.lib/_NEVSTOP/Communicable State Machine(CSM)/_popupMenuPlugin/_support/_Highlight CSM Scripts(TextDecor).vi", path "C:/Program Files (x86)/National Instruments/LabVIEW 2017/user.lib/_NEVSTOP/Communicable State Machine(CSM)/_popupMenuPlugin/_support/_Make String Safe as Arguments.vi", path "C:/Program Files (x86)/National Instruments/LabVIEW 2017/user.lib/_NEVSTOP/Communicable State Machine(CSM)/_popupMenuPlugin/_support/_Revert CSM Safe String.vi", path "C:/Program Files (x86)/National Instruments/LabVIEW 2017/user.lib/_NEVSTOP/Communicable State Machine(CSM)/_quickdrop/CSM - Flood of Events Handler Side Loop.vi", path "C:/Program Files (x86)/National Instruments/LabVIEW 2017/user.lib/_NEVSTOP/Communicable State Machine(CSM)/_quickdrop/CSM - Global Log Monitoring Loop.vi", path "C:/Program Files (x86)/National Instruments/LabVIEW 2017/user.lib/_NEVSTOP/Communicable State Machine(CSM)/_quickdrop/CSM - Start Async Call.vi", path "C:/Program Files (x86)/National Instruments/LabVIEW 2017/user.lib/_NEVSTOP/Communicable State Machine(CSM)/_quickdrop/CSM - Synchronized Call.vi", path "C:/Program Files (x86)/National Instruments/LabVIEW 2017/user.lib/_NEVSTOP/Communicable State Machine(CSM)/_quickdrop/CSM-QuickDrops.lvlib", path "C:/Program Files (x86)/National Instruments/LabVIEW 2017/user.lib/_NEVSTOP/Communicable State Machine(CSM)/_scripts/_csm_System_Language.vi", path "C:/Program Files (x86)/National Instruments/LabVIEW 2017/user.lib/_NEVSTOP/Communicable State Machine(CSM)/_scripts/_csm_user_lib_dir.vi", path "C:/Program Files (x86)/National Instruments/LabVIEW 2017/user.lib/_NEVSTOP/Communicable State Machine(CSM)/_scripts/_exclude Event Structure Ref.vi", path "C:/Program Files (x86)/National Instruments/LabVIEW 2017/user.lib/_NEVSTOP/Communicable State Machine(CSM)/_scripts/_script_add_vi_reference_case.vi", path "C:/Program Files (x86)/National Instruments/LabVIEW 2017/user.lib/_NEVSTOP/Communicable State Machine(CSM)/_scripts/_script_fix_jkism_helper.llb", path "C:/Program Files (x86)/National Instruments/LabVIEW 2017/user.lib/_NEVSTOP/Communicable State Machine(CSM)/_scripts/_script_remove_all_csm_bookmarks.vi", path "C:/Program Files (x86)/National Instruments/LabVIEW 2017/user.lib/_NEVSTOP/Communicable State Machine(CSM)/_scripts/_script_set_csm_doc_case_as_default.vi", path "C:/Program Files (x86)/National Instruments/LabVIEW 2017/user.lib/_NEVSTOP/Communicable State Machine(CSM)/_scripts/FixJKIHelper.vi", path "C:/Program Files (x86)/National Instruments/LabVIEW 2017/user.lib/_NEVSTOP/Communicable State Machine(CSM)/_scripts/sendkeys.bat", path "C:/Program Files (x86)/National Instruments/LabVIEW 2017/user.lib/_NEVSTOP/Communicable State Machine(CSM)/_scripts/_support/clear the mutation history for the classes.vi", path "C:/Program Files (x86)/National Instruments/LabVIEW 2017/user.lib/_NEVSTOP/Communicable State Machine(CSM)/_scripts/_support/CSM_Bookmarks_Refs.vi", path "C:/Program Files (x86)/National Instruments/LabVIEW 2017/user.lib/_NEVSTOP/Communicable State Machine(CSM)/_scripts/_support/is UTF-8_CSM.vi", path "C:/Program Files (x86)/National Instruments/LabVIEW 2017/user.lib/_NEVSTOP/Communicable State Machine(CSM)/_scripts/_support/load template description map.vi", path "C:/Program Files (x86)/National Instruments/LabVIEW 2017/user.lib/_NEVSTOP/Communicable State Machine(CSM)/_scripts/_support/Load TextConstant to md.vi", path "C:/Program Files (x86)/National Instruments/LabVIEW 2017/user.lib/_NEVSTOP/Communicable State Machine(CSM)/_scripts/_support/Operate_CSM_template_doc.vi", path "C:/Program Files (x86)/National Instruments/LabVIEW 2017/user.lib/_NEVSTOP/Communicable State Machine(CSM)/_scripts/_support/Periodic Trigger (OpenG).vi", path "C:/Program Files (x86)/National Instruments/LabVIEW 2017/user.lib/_NEVSTOP/Communicable State Machine(CSM)/_scripts/_support/Save TextConstant to md.vi", path "C:/Program Files (x86)/National Instruments/LabVIEW 2017/user.lib/_NEVSTOP/Communicable State Machine(CSM)/_scripts/_support/Split String Array By Patterns_CSM.vi", path "C:/Program Files (x86)/National Instruments/LabVIEW 2017/user.lib/_NEVSTOP/Communicable State Machine(CSM)/_scripts/_support/Text To Lines_CSM.vi", path "C:/Program Files (x86)/National Instruments/LabVIEW 2017/user.lib/_NEVSTOP/Communicable State Machine(CSM)/_scripts/_support/TxtFile Load_CSM.vi", path "C:/Program Files (x86)/National Instruments/LabVIEW 2017/user.lib/_NEVSTOP/Communicable State Machine(CSM)/_scripts/_support/BD teamplate/Case.vi", path "C:/Program Files (x86)/National Instruments/LabVIEW 2017/user.lib/_NEVSTOP/Communicable State Machine(CSM)/_scripts/_support/BD teamplate/Not a Num.vi", path "C:/Program Files (x86)/National Instruments/LabVIEW 2017/user.lib/_NEVSTOP/Communicable State Machine(CSM)/_scripts/_support/Constant String/Error Case Strings.vi", path "C:/Program Files (x86)/National Instruments/LabVIEW 2017/user.lib/_NEVSTOP/Communicable State Machine(CSM)/_scripts/_support/Constant String/Not a Num Primitive String.vi", path "C:/Program Files (x86)/National Instruments/LabVIEW 2017/user.lib/_NEVSTOP/Communicable State Machine(CSM)/_Support/CSM Dummy Module.vi", path "C:/Program Files (x86)/National Instruments/LabVIEW 2017/user.lib/_NEVSTOP/Communicable State Machine(CSM)/_Support/Def-CSMOMgr.ctl", path "C:/Program Files (x86)/National Instruments/LabVIEW 2017/user.lib/_NEVSTOP/Communicable State Machine(CSM)/_Support/Naming Check.vi", path "C:/Program Files (x86)/National Instruments/LabVIEW 2017/user.lib/_NEVSTOP/Communicable State Machine(CSM)/_Support/BroadcastRegistry/BroadcastRegistry.lvclass", path "C:/Program Files (x86)/National Instruments/LabVIEW 2017/user.lib/_NEVSTOP/Communicable State Machine(CSM)/_Support/BroadcastRegistry/Check.vi", path "C:/Program Files (x86)/National Instruments/LabVIEW 2017/user.lib/_NEVSTOP/Communicable State Machine(CSM)/_Support/BroadcastRegistry/Delete Source Module.vi", path "C:/Program Files (x86)/National Instruments/LabVIEW 2017/user.lib/_NEVSTOP/Communicable State Machine(CSM)/_Support/BroadcastRegistry/Delete Target Module.vi", path "C:/Program Files (x86)/National Instruments/LabVIEW 2017/user.lib/_NEVSTOP/Communicable State Machine(CSM)/_Support/BroadcastRegistry/Initialize.vi", path "C:/Program Files (x86)/National Instruments/LabVIEW 2017/user.lib/_NEVSTOP/Communicable State Machine(CSM)/_Support/BroadcastRegistry/List Entries.vi", path "C:/Program Files (x86)/National Instruments/LabVIEW 2017/user.lib/_NEVSTOP/Communicable State Machine(CSM)/_Support/BroadcastRegistry/List Status in Registry.vi", path "C:/Program Files (x86)/National Instruments/LabVIEW 2017/user.lib/_NEVSTOP/Communicable State Machine(CSM)/_Support/BroadcastRegistry/Register.vi", path "C:/Program Files (x86)/National Instruments/LabVIEW 2017/user.lib/_NEVSTOP/Communicable State Machine(CSM)/_Support/BroadcastRegistry/Remove Module.vi", path "C:/Program Files (x86)/National Instruments/LabVIEW 2017/user.lib/_NEVSTOP/Communicable State Machine(CSM)/_Support/BroadcastRegistry/Unregister.vi", path "C:/Program Files (x86)/National Instruments/LabVIEW 2017/user.lib/_NEVSTOP/Communicable State Machine(CSM)/_Support/BroadcastRegistry/HelperVI/Broadcast Item Key.vi", path "C:/Program Files (x86)/National Instruments/LabVIEW 2017/user.lib/_NEVSTOP/Communicable State Machine(CSM)/_Support/BroadcastRegistry/HelperVI/Preview.vi", path "C:/Program Files (x86)/National Instruments/LabVIEW 2017/user.lib/_NEVSTOP/Communicable State Machine(CSM)/_Support/BroadcastRegistry/HelperVI/Remove response API from List.vi", path "C:/Program Files (x86)/National Instruments/LabVIEW 2017/user.lib/_NEVSTOP/Communicable State Machine(CSM)/_Support/Common/Concatenate State with Arguments.vi", path "C:/Program Files (x86)/National Instruments/LabVIEW 2017/user.lib/_NEVSTOP/Communicable State Machine(CSM)/_Support/Common/CSM-Name to CSM-Mode.vi", path "C:/Program Files (x86)/National Instruments/LabVIEW 2017/user.lib/_NEVSTOP/Communicable State Machine(CSM)/_Support/Common/Format Timestamp.vi", path "C:/Program Files (x86)/National Instruments/LabVIEW 2017/user.lib/_NEVSTOP/Communicable State Machine(CSM)/_Support/Common/Hex Str to U8 Data.vi", path "C:/Program Files (x86)/National Instruments/LabVIEW 2017/user.lib/_NEVSTOP/Communicable State Machine(CSM)/_Support/Common/Parse Next Single-line State.vi", path "C:/Program Files (x86)/National Instruments/LabVIEW 2017/user.lib/_NEVSTOP/Communicable State Machine(CSM)/_Support/Common/Remove Comments from Line.vi", path "C:/Program Files (x86)/National Instruments/LabVIEW 2017/user.lib/_NEVSTOP/Communicable State Machine(CSM)/_Support/Common/Splite Reason String Part.vi", path "C:/Program Files (x86)/National Instruments/LabVIEW 2017/user.lib/_NEVSTOP/Communicable State Machine(CSM)/_Support/Common/Splite Single-line Message.vi", path "C:/Program Files (x86)/National Instruments/LabVIEW 2017/user.lib/_NEVSTOP/Communicable State Machine(CSM)/_Support/Common/Trim Single line Text.vi", path "C:/Program Files (x86)/National Instruments/LabVIEW 2017/user.lib/_NEVSTOP/Communicable State Machine(CSM)/_Support/Common/U8 Data to Hex Str.vi", path "C:/Program Files (x86)/National Instruments/LabVIEW 2017/user.lib/_NEVSTOP/Communicable State Machine(CSM)/_Support/CSMOMgr/CSMOMgr-Create CSMO.vi", path "C:/Program Files (x86)/National Instruments/LabVIEW 2017/user.lib/_NEVSTOP/Communicable State Machine(CSM)/_Support/CSMOMgr/CSMOMgr-Delete CSMO.vi", path "C:/Program Files (x86)/National Instruments/LabVIEW 2017/user.lib/_NEVSTOP/Communicable State Machine(CSM)/_Support/CSMOMgr/CSMOMgr-Duplication Check.vi", path "C:/Program Files (x86)/National Instruments/LabVIEW 2017/user.lib/_NEVSTOP/Communicable State Machine(CSM)/_Support/CSMOMgr/CSMOMgr-Get CSMO.vi", path "C:/Program Files (x86)/National Instruments/LabVIEW 2017/user.lib/_NEVSTOP/Communicable State Machine(CSM)/_Support/CSMOMgr/CSMOMgr-Update CSMO.vi", path "C:/Program Files (x86)/National Instruments/LabVIEW 2017/user.lib/_NEVSTOP/Communicable State Machine(CSM)/_Support/CSMQ/_Chain Mapping Map.vi", path "C:/Program Files (x86)/National Instruments/LabVIEW 2017/user.lib/_NEVSTOP/Communicable State Machine(CSM)/_Support/CSMQ/_CSMObj-Add Internal Registry Rule.vi", path "C:/Program Files (x86)/National Instruments/LabVIEW 2017/user.lib/_NEVSTOP/Communicable State Machine(CSM)/_Support/CSMQ/_CSMObj-Append Chain Node.vi", path "C:/Program Files (x86)/National Instruments/LabVIEW 2017/user.lib/_NEVSTOP/Communicable State Machine(CSM)/_Support/CSMQ/_CSMObj-Clone Worker.vi", path "C:/Program Files (x86)/National Instruments/LabVIEW 2017/user.lib/_NEVSTOP/Communicable State Machine(CSM)/_Support/CSMQ/_CSMObj-Create Status Event.vi", path "C:/Program Files (x86)/National Instruments/LabVIEW 2017/user.lib/_NEVSTOP/Communicable State Machine(CSM)/_Support/CSMQ/_CSMObj-Data.ctl", path "C:/Program Files (x86)/National Instruments/LabVIEW 2017/user.lib/_NEVSTOP/Communicable State Machine(CSM)/_Support/CSMQ/_CSMObj-Destroy Status Event.vi", path "C:/Program Files (x86)/National Instruments/LabVIEW 2017/user.lib/_NEVSTOP/Communicable State Machine(CSM)/_Support/CSMQ/_CSMObj-Enqueue Cross-Module Message.vi", path "C:/Program Files (x86)/National Instruments/LabVIEW 2017/user.lib/_NEVSTOP/Communicable State Machine(CSM)/_Support/CSMQ/_CSMObj-Lock State.vi", path "C:/Program Files (x86)/National Instruments/LabVIEW 2017/user.lib/_NEVSTOP/Communicable State Machine(CSM)/_Support/CSMQ/_CSMObj-Log Error if in a Remote Session.vi", path "C:/Program Files (x86)/National Instruments/LabVIEW 2017/user.lib/_NEVSTOP/Communicable State Machine(CSM)/_Support/CSMQ/_CSMObj-Message Check.vi", path "C:/Program Files (x86)/National Instruments/LabVIEW 2017/user.lib/_NEVSTOP/Communicable State Machine(CSM)/_Support/CSMQ/_CSMObj-ModeData.ctl", path "C:/Program Files (x86)/National Instruments/LabVIEW 2017/user.lib/_NEVSTOP/Communicable State Machine(CSM)/_Support/CSMQ/_CSMObj-Obtain Chain.vi", path "C:/Program Files (x86)/National Instruments/LabVIEW 2017/user.lib/_NEVSTOP/Communicable State Machine(CSM)/_Support/CSMQ/_CSMObj-Obtain.vi", path "C:/Program Files (x86)/National Instruments/LabVIEW 2017/user.lib/_NEVSTOP/Communicable State Machine(CSM)/_Support/CSMQ/_CSMObj-Release.vi", path "C:/Program Files (x86)/National Instruments/LabVIEW 2017/user.lib/_NEVSTOP/Communicable State Machine(CSM)/_Support/CSMQ/_CSMObj-Remove Chain Node.vi", path "C:/Program Files (x86)/National Instruments/LabVIEW 2017/user.lib/_NEVSTOP/Communicable State Machine(CSM)/_Support/CSMQ/_CSMObj-Remove Internal Registry Rule.vi", path "C:/Program Files (x86)/National Instruments/LabVIEW 2017/user.lib/_NEVSTOP/Communicable State Machine(CSM)/_Support/CSMQ/_CSMObj-Unlock.vi", path "C:/Program Files (x86)/National Instruments/LabVIEW 2017/user.lib/_NEVSTOP/Communicable State Machine(CSM)/_Support/CSMQ/_CSMObj-Unregister Internal Registry Rules.vi", path "C:/Program Files (x86)/National Instruments/LabVIEW 2017/user.lib/_NEVSTOP/Communicable State Machine(CSM)/_Support/CSMQ/_CSMObj.ctl", path "C:/Program Files (x86)/National Instruments/LabVIEW 2017/user.lib/_NEVSTOP/Communicable State Machine(CSM)/_Support/CSMQ/_CSMOFGV Dequeue.vi", path "C:/Program Files (x86)/National Instruments/LabVIEW 2017/user.lib/_NEVSTOP/Communicable State Machine(CSM)/_Support/CSMQ/_CSMOFGV Get.vi", path "C:/Program Files (x86)/National Instruments/LabVIEW 2017/user.lib/_NEVSTOP/Communicable State Machine(CSM)/_Support/CSMQ/_CSMOFGV Obtain.vi", path "C:/Program Files (x86)/National Instruments/LabVIEW 2017/user.lib/_NEVSTOP/Communicable State Machine(CSM)/_Support/CSMQ/_CSMOFGV Release.vi", path "C:/Program Files (x86)/National Instruments/LabVIEW 2017/user.lib/_NEVSTOP/Communicable State Machine(CSM)/_Support/CSMQ/_CSMOFGV.vi", path "C:/Program Files (x86)/National Instruments/LabVIEW 2017/user.lib/_NEVSTOP/Communicable State Machine(CSM)/_Support/CSMQ/_CSMOFGVOPER.ctl", path "C:/Program Files (x86)/National Instruments/LabVIEW 2017/user.lib/_NEVSTOP/Communicable State Machine(CSM)/_Support/CSMQ/_Obtain CSM Data Queue.vi", path "C:/Program Files (x86)/National Instruments/LabVIEW 2017/user.lib/_NEVSTOP/Communicable State Machine(CSM)/_Support/Error/CSM Critical Error.vi", path "C:/Program Files (x86)/National Instruments/LabVIEW 2017/user.lib/_NEVSTOP/Communicable State Machine(CSM)/_Support/Error/CSM No Target Error.vi", path "C:/Program Files (x86)/National Instruments/LabVIEW 2017/user.lib/_NEVSTOP/Communicable State Machine(CSM)/_Support/Error/CSM Not Allowed Message.vi", path "C:/Program Files (x86)/National Instruments/LabVIEW 2017/user.lib/_NEVSTOP/Communicable State Machine(CSM)/_Support/Error/CSM Target Error.vi", path "C:/Program Files (x86)/National Instruments/LabVIEW 2017/user.lib/_NEVSTOP/Communicable State Machine(CSM)/_Support/Error/CSM Target Timeout Error.vi", path "C:/Program Files (x86)/National Instruments/LabVIEW 2017/user.lib/_NEVSTOP/Communicable State Machine(CSM)/_Support/Error/CSM Unhandled State Error.vi", path "C:/Program Files (x86)/National Instruments/LabVIEW 2017/user.lib/_NEVSTOP/Communicable State Machine(CSM)/_Support/FGV-BroadcastRegistry/Cache-Broadcast Registry Search Result.vi", path "C:/Program Files (x86)/National Instruments/LabVIEW 2017/user.lib/_NEVSTOP/Communicable State Machine(CSM)/_Support/FGV-BroadcastRegistry/FGV-BroadcastRegistry.vi", path "C:/Program Files (x86)/National Instruments/LabVIEW 2017/user.lib/_NEVSTOP/Communicable State Machine(CSM)/_Support/FGV-BroadcastRegistry/global-Broadcast Cache Change Flag.vi", path "C:/Program Files (x86)/National Instruments/LabVIEW 2017/user.lib/_NEVSTOP/Communicable State Machine(CSM)/_Support/FGV-BroadcastRegistry/global-CSMQ FGV Change Flag.vi", path "C:/Program Files (x86)/National Instruments/LabVIEW 2017/user.lib/_NEVSTOP/Communicable State Machine(CSM)/_Support/FGV-BroadcastRegistry/Operation-BroadcastRegistry.ctl", path "C:/Program Files (x86)/National Instruments/LabVIEW 2017/user.lib/_NEVSTOP/Communicable State Machine(CSM)/_Support/GlobalEvent/Cache-GEvt Filter Object.vi", path "C:/Program Files (x86)/National Instruments/LabVIEW 2017/user.lib/_NEVSTOP/Communicable State Machine(CSM)/_Support/GlobalEvent/FGV-GEvt Filter Obj.vi", path "C:/Program Files (x86)/National Instruments/LabVIEW 2017/user.lib/_NEVSTOP/Communicable State Machine(CSM)/_Support/GlobalEvent/FGV-GlobalEventRef.vi", path "C:/Program Files (x86)/National Instruments/LabVIEW 2017/user.lib/_NEVSTOP/Communicable State Machine(CSM)/_Support/GlobalEvent/FGV-StatusChangeEventRef.vi", path "C:/Program Files (x86)/National Instruments/LabVIEW 2017/user.lib/_NEVSTOP/Communicable State Machine(CSM)/_Support/GlobalEvent/GEvt-BackgroundThread.vi", path "C:/Program Files (x86)/National Instruments/LabVIEW 2017/user.lib/_NEVSTOP/Communicable State Machine(CSM)/_Support/GlobalEvent/GEvt-Convert Filter Rules - Periodic Setting Only.vi", path "C:/Program Files (x86)/National Instruments/LabVIEW 2017/user.lib/_NEVSTOP/Communicable State Machine(CSM)/_Support/GlobalEvent/GEvt-Convert Filter Rules - v1.0.vi", path "C:/Program Files (x86)/National Instruments/LabVIEW 2017/user.lib/_NEVSTOP/Communicable State Machine(CSM)/_Support/GlobalEvent/GEvt-Convert Filter Rules - v1.1.vi", path "C:/Program Files (x86)/National Instruments/LabVIEW 2017/user.lib/_NEVSTOP/Communicable State Machine(CSM)/_Support/GlobalEvent/GEvt-Filter Global Log - v1.0.vi", path "C:/Program Files (x86)/National Instruments/LabVIEW 2017/user.lib/_NEVSTOP/Communicable State Machine(CSM)/_Support/GlobalEvent/GEvt-Filter Global Log - v1.1.vi", path "C:/Program Files (x86)/National Instruments/LabVIEW 2017/user.lib/_NEVSTOP/Communicable State Machine(CSM)/_Support/GlobalEvent/GEvt-Generate Complete Log.vi", path "C:/Program Files (x86)/National Instruments/LabVIEW 2017/user.lib/_NEVSTOP/Communicable State Machine(CSM)/_Support/GlobalEvent/GEvt-Generate Interrupt Log.vi", path "C:/Program Files (x86)/National Instruments/LabVIEW 2017/user.lib/_NEVSTOP/Communicable State Machine(CSM)/_Support/GlobalEvent/GEvt-Generate Module Created Log.vi", path "C:/Program Files (x86)/National Instruments/LabVIEW 2017/user.lib/_NEVSTOP/Communicable State Machine(CSM)/_Support/GlobalEvent/GEvt-Generate Module Destroyed Log.vi", path "C:/Program Files (x86)/National Instruments/LabVIEW 2017/user.lib/_NEVSTOP/Communicable State Machine(CSM)/_Support/GlobalEvent/GEvt-Generate Register Log.vi", path "C:/Program Files (x86)/National Instruments/LabVIEW 2017/user.lib/_NEVSTOP/Communicable State Machine(CSM)/_Support/GlobalEvent/GEvt-Generate Remaining States Log.vi", path "C:/Program Files (x86)/National Instruments/LabVIEW 2017/user.lib/_NEVSTOP/Communicable State Machine(CSM)/_Support/GlobalEvent/GEvt-Generate State Change Log.vi", path "C:/Program Files (x86)/National Instruments/LabVIEW 2017/user.lib/_NEVSTOP/Communicable State Machine(CSM)/_Support/GlobalEvent/GEvt-Generate Status Log.vi", path "C:/Program Files (x86)/National Instruments/LabVIEW 2017/user.lib/_NEVSTOP/Communicable State Machine(CSM)/_Support/GlobalEvent/GEvt-Generate Unregister Log.vi", path "C:/Program Files (x86)/National Instruments/LabVIEW 2017/user.lib/_NEVSTOP/Communicable State Machine(CSM)/_Support/GlobalEvent/GEvt-Generate with Rule Check.vi", path "C:/Program Files (x86)/National Instruments/LabVIEW 2017/user.lib/_NEVSTOP/Communicable State Machine(CSM)/_Support/GlobalEvent/GEvt-RequestDef.ctl", path "C:/Program Files (x86)/National Instruments/LabVIEW 2017/user.lib/_NEVSTOP/Communicable State Machine(CSM)/_Support/GlobalEvent/GEvt-Set Source Filter Rules - v1.0.vi", path "C:/Program Files (x86)/National Instruments/LabVIEW 2017/user.lib/_NEVSTOP/Communicable State Machine(CSM)/_Support/GlobalEvent/Gevt-ThreadQueueName.vi", path "C:/Program Files (x86)/National Instruments/LabVIEW 2017/user.lib/_NEVSTOP/Communicable State Machine(CSM)/_Support/GlobalEvent/GEvt-WatchdogThread.vi", path "C:/Program Files (x86)/National Instruments/LabVIEW 2017/user.lib/_NEVSTOP/Communicable State Machine(CSM)/_Support/GlobalEvent/global-GEvnt Filter Change Flag.vi", path "C:/Program Files (x86)/National Instruments/LabVIEW 2017/user.lib/_NEVSTOP/Communicable State Machine(CSM)/_Support/GlobalEvent/LogFilter/LogFilter - Check.vi", path "C:/Program Files (x86)/National Instruments/LabVIEW 2017/user.lib/_NEVSTOP/Communicable State Machine(CSM)/_Support/GlobalEvent/LogFilter/LogFilter - Periodic Log Check.vi", path "C:/Program Files (x86)/National Instruments/LabVIEW 2017/user.lib/_NEVSTOP/Communicable State Machine(CSM)/_Support/GlobalEvent/LogFilter/LogFilter.lvclass", path "C:/Program Files (x86)/National Instruments/LabVIEW 2017/user.lib/_NEVSTOP/Communicable State Machine(CSM)/_Support/GlobalEvent/LogFilter/Periodic Log Filter Check2.vi", path "C:/Program Files (x86)/National Instruments/LabVIEW 2017/user.lib/_NEVSTOP/Communicable State Machine(CSM)/_Support/GlobalEvent/LogFilter/CheckVIs/CSM Check - LogType.vi", path "C:/Program Files (x86)/National Instruments/LabVIEW 2017/user.lib/_NEVSTOP/Communicable State Machine(CSM)/_Support/GlobalEvent/LogFilter/CheckVIs/CSM Check - State.vi", path "C:/Program Files (x86)/National Instruments/LabVIEW 2017/user.lib/_NEVSTOP/Communicable State Machine(CSM)/_Support/GlobalEvent/LogFilter/CheckVIs/CSM Check - StateType.vi", path "C:/Program Files (x86)/National Instruments/LabVIEW 2017/user.lib/_NEVSTOP/Communicable State Machine(CSM)/_Support/GlobalEvent/LogFilter/CheckVIs/Group Check - CSM.vi", path "C:/Program Files (x86)/National Instruments/LabVIEW 2017/user.lib/_NEVSTOP/Communicable State Machine(CSM)/_Support/GlobalEvent/LogFilter/CheckVIs/Group Check - LogType.vi", path "C:/Program Files (x86)/National Instruments/LabVIEW 2017/user.lib/_NEVSTOP/Communicable State Machine(CSM)/_Support/GlobalEvent/LogFilter/CheckVIs/Group Check - State.vi", path "C:/Program Files (x86)/National Instruments/LabVIEW 2017/user.lib/_NEVSTOP/Communicable State Machine(CSM)/_Support/GlobalEvent/LogFilter/CheckVIs/Group Check - StateType.vi", path "C:/Program Files (x86)/National Instruments/LabVIEW 2017/user.lib/_NEVSTOP/Communicable State Machine(CSM)/_Support/GlobalEvent/LogFilter/CheckVIs/Periodic Log Filter Check.vi", path "C:/Program Files (x86)/National Instruments/LabVIEW 2017/user.lib/_NEVSTOP/Communicable State Machine(CSM)/_Support/GlobalEvent/LogFilter/SettingVIs/Read Rules.vi", path "C:/Program Files (x86)/National Instruments/LabVIEW 2017/user.lib/_NEVSTOP/Communicable State Machine(CSM)/_Support/GlobalEvent/LogFilter/SettingVIs/Set CSM LogType Filter.vi", path "C:/Program Files (x86)/National Instruments/LabVIEW 2017/user.lib/_NEVSTOP/Communicable State Machine(CSM)/_Support/GlobalEvent/LogFilter/SettingVIs/Set CSM State Filter.vi", path "C:/Program Files (x86)/National Instruments/LabVIEW 2017/user.lib/_NEVSTOP/Communicable State Machine(CSM)/_Support/GlobalEvent/LogFilter/SettingVIs/Set CSM StateType Filter.vi", path "C:/Program Files (x86)/National Instruments/LabVIEW 2017/user.lib/_NEVSTOP/Communicable State Machine(CSM)/_Support/GlobalEvent/LogFilter/SettingVIs/Set Global CSM Filter.vi", path "C:/Program Files (x86)/National Instruments/LabVIEW 2017/user.lib/_NEVSTOP/Communicable State Machine(CSM)/_Support/GlobalEvent/LogFilter/SettingVIs/Set Global LogType Filter.vi", path "C:/Program Files (x86)/National Instruments/LabVIEW 2017/user.lib/_NEVSTOP/Communicable State Machine(CSM)/_Support/GlobalEvent/LogFilter/SettingVIs/Set Global State Filter.vi", path "C:/Program Files (x86)/National Instruments/LabVIEW 2017/user.lib/_NEVSTOP/Communicable State Machine(CSM)/_Support/GlobalEvent/LogFilter/SettingVIs/Set Global StateType Filter.vi", path "C:/Program Files (x86)/National Instruments/LabVIEW 2017/user.lib/_NEVSTOP/Communicable State Machine(CSM)/_Support/GlobalEvent/LogFilter/SettingVIs/Set Periodic Log Filter.vi", path "C:/Program Files (x86)/National Instruments/LabVIEW 2017/user.lib/_NEVSTOP/Communicable State Machine(CSM)/_Support/GlobalEvent/LogFilter/Support/Log State Type.vi", path "C:/Program Files (x86)/National Instruments/LabVIEW 2017/user.lib/_NEVSTOP/Communicable State Machine(CSM)/_Support/Message/Parse Register Message.vi", path "C:/Program Files (x86)/National Instruments/LabVIEW 2017/user.lib/_NEVSTOP/Communicable State Machine(CSM)/_Support/Message/Parse State with Arguments String.vi", path "C:/Program Files (x86)/National Instruments/LabVIEW 2017/user.lib/_NEVSTOP/Communicable State Machine(CSM)/_Support/Message/Parse Unregister Message.vi", path "C:/Program Files (x86)/National Instruments/LabVIEW 2017/user.lib/_NEVSTOP/Communicable State Machine(CSM)/_Support/Priority Queue/def-Data(LowPRI-Q).ctl", path "C:/Program Files (x86)/National Instruments/LabVIEW 2017/user.lib/_NEVSTOP/Communicable State Machine(CSM)/_Support/Priority Queue/Dequeue Element.vi", path "C:/Program Files (x86)/National Instruments/LabVIEW 2017/user.lib/_NEVSTOP/Communicable State Machine(CSM)/_Support/Priority Queue/Enqueue Element.vi", path "C:/Program Files (x86)/National Instruments/LabVIEW 2017/user.lib/_NEVSTOP/Communicable State Machine(CSM)/_Support/Priority Queue/Get Queue Status.vi", path "C:/Program Files (x86)/National Instruments/LabVIEW 2017/user.lib/_NEVSTOP/Communicable State Machine(CSM)/_Support/Priority Queue/Not a Refnum.vi", path "C:/Program Files (x86)/National Instruments/LabVIEW 2017/user.lib/_NEVSTOP/Communicable State Machine(CSM)/_Support/Priority Queue/Obtain Priority Queue.vi", path "C:/Program Files (x86)/National Instruments/LabVIEW 2017/user.lib/_NEVSTOP/Communicable State Machine(CSM)/_Support/Priority Queue/Priority Queue.lvclass", path "C:/Program Files (x86)/National Instruments/LabVIEW 2017/user.lib/_NEVSTOP/Communicable State Machine(CSM)/_Support/Priority Queue/Release Priority Queue.vi", path "C:/Program Files (x86)/National Instruments/LabVIEW 2017/user.lib/_NEVSTOP/Communicable State Machine(CSM)/_Support/Process/CSMP-Async Call.vi", path "C:/Program Files (x86)/National Instruments/LabVIEW 2017/user.lib/_NEVSTOP/Communicable State Machine(CSM)/_Support/Process/CSMP-Broadcast.vi", path "C:/Program Files (x86)/National Instruments/LabVIEW 2017/user.lib/_NEVSTOP/Communicable State Machine(CSM)/_Support/Process/CSMP-PostPostMsg.vi", path "C:/Program Files (x86)/National Instruments/LabVIEW 2017/user.lib/_NEVSTOP/Communicable State Machine(CSM)/_Support/Process/CSMP-PostSendMsg.vi", path "C:/Program Files (x86)/National Instruments/LabVIEW 2017/user.lib/_NEVSTOP/Communicable State Machine(CSM)/_Support/Process/CSMP-Register Status.vi", path "C:/Program Files (x86)/National Instruments/LabVIEW 2017/user.lib/_NEVSTOP/Communicable State Machine(CSM)/_Support/Process/CSMP-Sync Call.vi", path "C:/Program Files (x86)/National Instruments/LabVIEW 2017/user.lib/_NEVSTOP/Communicable State Machine(CSM)/_Support/Process/CSMP-Unregister Status.vi", path "C:/Program Files (x86)/National Instruments/LabVIEW 2017/user.lib/_NEVSTOP/Communicable State Machine(CSM)/_Support/Typedef/_Cross CSM State Data.ctl", path "C:/Program Files (x86)/National Instruments/LabVIEW 2017/user.lib/_NEVSTOP/Communicable State Machine(CSM)/_Support/Typedef/_Cross CSM State Response.ctl", path "C:/Program Files (x86)/National Instruments/LabVIEW 2017/user.lib/_NEVSTOP/Communicable State Machine(CSM)/_Support/Typedef/_CSM Status Change Event Data.ctl", path "C:/Program Files (x86)/National Instruments/LabVIEW 2017/user.lib/_NEVSTOP/Communicable State Machine(CSM)/_Support/Typedef/_CSM_Broadcast_Response_Message_info.ctl", path "C:/Program Files (x86)/National Instruments/LabVIEW 2017/user.lib/_NEVSTOP/Communicable State Machine(CSM)/_Support/Typedef/_CSM_GlobalLog Filter Rules - v1.0.ctl", path "C:/Program Files (x86)/National Instruments/LabVIEW 2017/user.lib/_NEVSTOP/Communicable State Machine(CSM)/_Support/Typedef/_CSM_GlobalLog Filter Rules - v1.1.ctl", path "C:/Program Files (x86)/National Instruments/LabVIEW 2017/user.lib/_NEVSTOP/Communicable State Machine(CSM)/_Support/Typedef/_CSM_GlobalLog_MSG.ctl", path "C:/Program Files (x86)/National Instruments/LabVIEW 2017/user.lib/_NEVSTOP/Communicable State Machine(CSM)/_Support/Typedef/_CSM_GlobalLog_MSG_TYPE.ctl", path "C:/Program Files (x86)/National Instruments/LabVIEW 2017/user.lib/_NEVSTOP/Communicable State Machine(CSM)/_Support/Typedef/_CSM_GlobalLog_STATE_TYPE.ctl", path "C:/Program Files (x86)/National Instruments/LabVIEW 2017/user.lib/_NEVSTOP/Communicable State Machine(CSM)/_Support/Typedef/_CSM_MODE.ctl", path "C:/Program Files (x86)/National Instruments/LabVIEW 2017/user.lib/_NEVSTOP/Communicable State Machine(CSM)/_Support/Typedef/_CSM_MSG_TYPE.ctl", path "C:/Program Files (x86)/National Instruments/LabVIEW 2017/user.lib/_NEVSTOP/Communicable State Machine(CSM)/_Support/Typedef/_CSM_NAME_REQUEST.ctl", path "C:/Program Files (x86)/National Instruments/LabVIEW 2017/user.lib/_NEVSTOP/Communicable State Machine(CSM)/_Support/Typedef/_CSM_Response Source Message.ctl", path "C:/Program Files (x86)/National Instruments/LabVIEW 2017/user.lib/_NEVSTOP/Communicable State Machine(CSM)/_tool/CSM - Add VI Reference Case to CSMs.vi", path "C:/Program Files (x86)/National Instruments/LabVIEW 2017/user.lib/_NEVSTOP/Communicable State Machine(CSM)/_tool/CSM - Debug Console - DebugTool.vi", path "C:/Program Files (x86)/National Instruments/LabVIEW 2017/user.lib/_NEVSTOP/Communicable State Machine(CSM)/_tool/CSM - Remove all CSM Bookmarks.vi", path "C:/Program Files (x86)/National Instruments/LabVIEW 2017/user.lib/_NEVSTOP/Communicable State Machine(CSM)/_tool/CSM - Running Log - DebugTool.vi", path "C:/Program Files (x86)/National Instruments/LabVIEW 2017/user.lib/_NEVSTOP/Communicable State Machine(CSM)/_tool/CSM - State Dashboard - DebugTool.vi", path "C:/Program Files (x86)/National Instruments/LabVIEW 2017/user.lib/_NEVSTOP/Communicable State Machine(CSM)/_tool/CSM - State Table - DebugTool.vi", path "C:/Program Files (x86)/National Instruments/LabVIEW 2017/user.lib/_NEVSTOP/Communicable State Machine(CSM)/_tool/CSM - Switch Language Tool.vi", path "C:/Program Files (x86)/National Instruments/LabVIEW 2017/user.lib/_NEVSTOP/Communicable State Machine(CSM)/_tool/_backup/Script - JKISM to CSM.vi", path "C:/Program Files (x86)/National Instruments/LabVIEW 2017/user.lib/_NEVSTOP/Communicable State Machine(CSM)/_tool/_jksm/Destroy JKISM Message Event.vi", path "C:/Program Files (x86)/National Instruments/LabVIEW 2017/user.lib/_NEVSTOP/Communicable State Machine(CSM)/_tool/_jksm/Generate JKISM Message Event.vi", path "C:/Program Files (x86)/National Instruments/LabVIEW 2017/user.lib/_NEVSTOP/Communicable State Machine(CSM)/_tool/_jksm/JKISM Message Event.lvlib", path "C:/Program Files (x86)/National Instruments/LabVIEW 2017/user.lib/_NEVSTOP/Communicable State Machine(CSM)/_tool/_jksm/Obtain JKISM Message Event.vi", path "C:/Program Files (x86)/National Instruments/LabVIEW 2017/user.lib/_NEVSTOP/Communicable State Machine(CSM)/_tool/_SubModules/_CSM Message Communication Panel.vi", path "C:/Program Files (x86)/National Instruments/LabVIEW 2017/user.lib/_NEVSTOP/Communicable State Machine(CSM)/_tool/_SubModules/_CSM Module Switcher.vi", path "C:/Program Files (x86)/National Instruments/LabVIEW 2017/user.lib/_NEVSTOP/Communicable State Machine(CSM)/_tool/_Support/Auto Resize All MultiListbox Columns (Uniform Text).vi", path "C:/Program Files (x86)/National Instruments/LabVIEW 2017/user.lib/_NEVSTOP/Communicable State Machine(CSM)/_tool/_Support/csm-tool-support.lvlib", path "C:/Program Files (x86)/National Instruments/LabVIEW 2017/user.lib/_NEVSTOP/Communicable State Machine(CSM)/_tool/_Support/Dashboard Cell Resize.vi", path "C:/Program Files (x86)/National Instruments/LabVIEW 2017/user.lib/_NEVSTOP/Communicable State Machine(CSM)/_tool/_Support/Dashboard Cell2 Array Resize.vi", path "C:/Program Files (x86)/National Instruments/LabVIEW 2017/user.lib/_NEVSTOP/Communicable State Machine(CSM)/_tool/_Support/Open CSM BD.vi", path "C:/Program Files (x86)/National Instruments/LabVIEW 2017/user.lib/_NEVSTOP/Communicable State Machine(CSM)/_tool/_Support/Open CSM FP.vi", path "C:/Program Files (x86)/National Instruments/LabVIEW 2017/user.lib/_NEVSTOP/Communicable State Machine(CSM)/_tool/_Support/Select Greater_nevstop.vi", path "C:/Program Files (x86)/National Instruments/LabVIEW 2017/user.lib/_NEVSTOP/Communicable State Machine(CSM)/_xnode/browse_nevstoplab/CSM - Explorer to Example.xnode", path "C:/Program Files (x86)/National Instruments/LabVIEW 2017/user.lib/_NEVSTOP/Communicable State Machine(CSM)/_xnode/browse_nevstoplab/_xnode_browse_nevstoplab_support/_Copy 1.vi", path "C:/Program Files (x86)/National Instruments/LabVIEW 2017/user.lib/_NEVSTOP/Communicable State Machine(CSM)/_xnode/browse_nevstoplab/_xnode_browse_nevstoplab_support/_GetHelp 1.vi", path "C:/Program Files (x86)/National Instruments/LabVIEW 2017/user.lib/_NEVSTOP/Communicable State Machine(CSM)/_xnode/browse_nevstoplab/_xnode_browse_nevstoplab_support/_Open Explorer Window.vi", path "C:/Program Files (x86)/National Instruments/LabVIEW 2017/user.lib/_NEVSTOP/Communicable State Machine(CSM)/_xnode/browse_nevstoplab/_xnode_browse_nevstoplab_support/_State 1.ctl", path "C:/Program Files (x86)/National Instruments/LabVIEW 2017/user.lib/_NEVSTOP/Communicable State Machine(CSM)/_xnode/csm_tool/CSM - DebugTool.xnode", path "C:/Program Files (x86)/National Instruments/LabVIEW 2017/user.lib/_NEVSTOP/Communicable State Machine(CSM)/_xnode/csm_tool/_xnode_csm_tool_support/_Copy 1.vi", path "C:/Program Files (x86)/National Instruments/LabVIEW 2017/user.lib/_NEVSTOP/Communicable State Machine(CSM)/_xnode/csm_tool/_xnode_csm_tool_support/_GetHelp 1.vi", path "C:/Program Files (x86)/National Instruments/LabVIEW 2017/user.lib/_NEVSTOP/Communicable State Machine(CSM)/_xnode/csm_tool/_xnode_csm_tool_support/_reorder tool entries.vi", path "C:/Program Files (x86)/National Instruments/LabVIEW 2017/user.lib/_NEVSTOP/Communicable State Machine(CSM)/_xnode/csm_tool/_xnode_csm_tool_support/_State 1.ctl", path "C:/Program Files (x86)/National Instruments/LabVIEW 2017/user.lib/_NEVSTOP/Communicable State Machine(CSM)/_xnode/csm_tool/_xnode_csm_tool_support/CSM DebugTool Dialog Ref(FGV).vi", path "C:/Program Files (x86)/National Instruments/LabVIEW 2017/user.lib/_NEVSTOP/Communicable State Machine(CSM)/_xnode/csm_tool/_xnode_csm_tool_support/CSM DebugTool Dialog.vi", path "C:/Program Files (x86)/National Instruments/LabVIEW 2017/user.lib/_NEVSTOP/Communicable State Machine(CSM)/_xnode/csm_tool/_xnode_csm_tool_support/Start CSM DebugTool Dialog.vi", path "C:/Program Files (x86)/National Instruments/LabVIEW 2017/user.lib/_NEVSTOP/Communicable State Machine(CSM)/addons/dir.mnu", path "C:/Program Files (x86)/National Instruments/LabVIEW 2017/user.lib/_NEVSTOP/Communicable State Machine(CSM)/addons/API-String-Arugments-Support/API String - Add Boolean Strings.vi", path "C:/Program Files (x86)/National Instruments/LabVIEW 2017/user.lib/_NEVSTOP/Communicable State Machine(CSM)/addons/API-String-Arugments-Support/API String - Float Format String.vi", path "C:/Program Files (x86)/National Instruments/LabVIEW 2017/user.lib/_NEVSTOP/Communicable State Machine(CSM)/addons/API-String-Arugments-Support/API String - List Boolean Strings.vi", path "C:/Program Files (x86)/National Instruments/LabVIEW 2017/user.lib/_NEVSTOP/Communicable State Machine(CSM)/addons/API-String-Arugments-Support/API String - Remove Boolean Strings.vi", path "C:/Program Files (x86)/National Instruments/LabVIEW 2017/user.lib/_NEVSTOP/Communicable State Machine(CSM)/addons/API-String-Arugments-Support/API String - Set Float Format String.vi", path "C:/Program Files (x86)/National Instruments/LabVIEW 2017/user.lib/_NEVSTOP/Communicable State Machine(CSM)/addons/API-String-Arugments-Support/API String - Set Float Precision.vi", path "C:/Program Files (x86)/National Instruments/LabVIEW 2017/user.lib/_NEVSTOP/Communicable State Machine(CSM)/addons/API-String-Arugments-Support/API String Arguments Support.lvlib", path "C:/Program Files (x86)/National Instruments/LabVIEW 2017/user.lib/_NEVSTOP/Communicable State Machine(CSM)/addons/API-String-Arugments-Support/Configure.mnu", path "C:/Program Files (x86)/National Instruments/LabVIEW 2017/user.lib/_NEVSTOP/Communicable State Machine(CSM)/addons/API-String-Arugments-Support/Convert API String Arguments to Data.vim", path "C:/Program Files (x86)/National Instruments/LabVIEW 2017/user.lib/_NEVSTOP/Communicable State Machine(CSM)/addons/API-String-Arugments-Support/Convert Data To API String Arguments.vim", path "C:/Program Files (x86)/National Instruments/LabVIEW 2017/user.lib/_NEVSTOP/Communicable State Machine(CSM)/addons/API-String-Arugments-Support/CSM - Broadcast Data As API String.vim", path "C:/Program Files (x86)/National Instruments/LabVIEW 2017/user.lib/_NEVSTOP/Communicable State Machine(CSM)/addons/API-String-Arugments-Support/CSM - Convert HexStr to Data.vim", path "C:/Program Files (x86)/National Instruments/LabVIEW 2017/user.lib/_NEVSTOP/Communicable State Machine(CSM)/addons/API-String-Arugments-Support/CSM - Module VI Ref.vi", path "C:/Program Files (x86)/National Instruments/LabVIEW 2017/user.lib/_NEVSTOP/Communicable State Machine(CSM)/addons/API-String-Arugments-Support/CSM - Query CSM VI Ref By API String.vi", path "C:/Program Files (x86)/National Instruments/LabVIEW 2017/user.lib/_NEVSTOP/Communicable State Machine(CSM)/addons/API-String-Arugments-Support/CSM - Query Internal Data Names By API String.vi", path "C:/Program Files (x86)/National Instruments/LabVIEW 2017/user.lib/_NEVSTOP/Communicable State Machine(CSM)/addons/API-String-Arugments-Support/CSM - Timestamp to API String Arguments.vi", path "C:/Program Files (x86)/National Instruments/LabVIEW 2017/user.lib/_NEVSTOP/Communicable State Machine(CSM)/addons/API-String-Arugments-Support/CSM-Utility.mnu", path "C:/Program Files (x86)/National Instruments/LabVIEW 2017/user.lib/_NEVSTOP/Communicable State Machine(CSM)/addons/API-String-Arugments-Support/dir.mnu", path "C:/Program Files (x86)/National Instruments/LabVIEW 2017/user.lib/_NEVSTOP/Communicable State Machine(CSM)/addons/API-String-Arugments-Support/Query Data as API String Arguments.vim", path "C:/Program Files (x86)/National Instruments/LabVIEW 2017/user.lib/_NEVSTOP/Communicable State Machine(CSM)/addons/API-String-Arugments-Support/Utility.mnu", path "C:/Program Files (x86)/National Instruments/LabVIEW 2017/user.lib/_NEVSTOP/Communicable State Machine(CSM)/addons/API-String-Arugments-Support/_Support/API String to 1D Array.vi", path "C:/Program Files (x86)/National Instruments/LabVIEW 2017/user.lib/_NEVSTOP/Communicable State Machine(CSM)/addons/API-String-Arugments-Support/_Support/Boolean Strings.vi", path "C:/Program Files (x86)/National Instruments/LabVIEW 2017/user.lib/_NEVSTOP/Communicable State Machine(CSM)/addons/API-String-Arugments-Support/_Support/Cluster API String to 1D Array(Splite Nested Cluster).vi", path "C:/Program Files (x86)/National Instruments/LabVIEW 2017/user.lib/_NEVSTOP/Communicable State Machine(CSM)/addons/API-String-Arugments-Support/_Support/Compare Two Numbers_csm.vim", path "C:/Program Files (x86)/National Instruments/LabVIEW 2017/user.lib/_NEVSTOP/Communicable State Machine(CSM)/addons/API-String-Arugments-Support/_Support/Concatenate Strings If not Empty_csm.vi", path "C:/Program Files (x86)/National Instruments/LabVIEW 2017/user.lib/_NEVSTOP/Communicable State Machine(CSM)/addons/API-String-Arugments-Support/_Support/Convert API String Arguments to Data(variant).vi", path "C:/Program Files (x86)/National Instruments/LabVIEW 2017/user.lib/_NEVSTOP/Communicable State Machine(CSM)/addons/API-String-Arugments-Support/_Support/Data To API String Arguments.vi", path "C:/Program Files (x86)/National Instruments/LabVIEW 2017/user.lib/_NEVSTOP/Communicable State Machine(CSM)/addons/API-String-Arugments-Support/_Support/Data To SingleElementsArray_csm.vi", path "C:/Program Files (x86)/National Instruments/LabVIEW 2017/user.lib/_NEVSTOP/Communicable State Machine(CSM)/addons/API-String-Arugments-Support/_Support/Data To SingleElementsArray_with_itself_csm.vi", path "C:/Program Files (x86)/National Instruments/LabVIEW 2017/user.lib/_NEVSTOP/Communicable State Machine(CSM)/addons/API-String-Arugments-Support/_Support/Float Precision.vi", path "C:/Program Files (x86)/National Instruments/LabVIEW 2017/user.lib/_NEVSTOP/Communicable State Machine(CSM)/addons/API-String-Arugments-Support/_Support/Indexed Enum to Numeric_csm.vim", path "C:/Program Files (x86)/National Instruments/LabVIEW 2017/user.lib/_NEVSTOP/Communicable State Machine(CSM)/addons/API-String-Arugments-Support/_Support/Indexed String To Enum_csm.vi", path "C:/Program Files (x86)/National Instruments/LabVIEW 2017/user.lib/_NEVSTOP/Communicable State Machine(CSM)/addons/API-String-Arugments-Support/_Support/Match Multiple Pattern_csm.vi", path "C:/Program Files (x86)/National Instruments/LabVIEW 2017/user.lib/_NEVSTOP/Communicable State Machine(CSM)/addons/API-String-Arugments-Support/_Support/Numeric to Indexed Enum_csm.vim", path "C:/Program Files (x86)/National Instruments/LabVIEW 2017/user.lib/_NEVSTOP/Communicable State Machine(CSM)/addons/API-String-Arugments-Support/_Support/Query Data as API String Arguments(variant).vi", path "C:/Program Files (x86)/National Instruments/LabVIEW 2017/user.lib/_NEVSTOP/Communicable State Machine(CSM)/addons/API-String-Arugments-Support/_Support/SingleElementsArray To Data_csm.vi", path "C:/Program Files (x86)/National Instruments/LabVIEW 2017/user.lib/_NEVSTOP/Communicable State Machine(CSM)/addons/API-String-Arugments-Support/_Support/String to Boolean_csm.vi", path "C:/Program Files (x86)/National Instruments/LabVIEW 2017/user.lib/_NEVSTOP/Communicable State Machine(CSM)/addons/API-String-Arugments-Support/_Support/String To Float_csm.vi", path "C:/Program Files (x86)/National Instruments/LabVIEW 2017/user.lib/_NEVSTOP/Communicable State Machine(CSM)/addons/API-String-Arugments-Support/_Support/String To Indexed Enum_csm.vi", path "C:/Program Files (x86)/National Instruments/LabVIEW 2017/user.lib/_NEVSTOP/Communicable State Machine(CSM)/addons/API-String-Arugments-Support/_Support/String To Number(I64)_csm.vi", path "C:/Program Files (x86)/National Instruments/LabVIEW 2017/user.lib/_NEVSTOP/Communicable State Machine(CSM)/addons/API-String-Arugments-Support/_Support/Strip Tag in Tag Value Pair.vi", path "C:/Program Files (x86)/National Instruments/LabVIEW 2017/user.lib/_NEVSTOP/Communicable State Machine(CSM)/addons/API-String-Arugments-Support/_Support/StringAnalyze/bracket code.vi", path "C:/Program Files (x86)/National Instruments/LabVIEW 2017/user.lib/_NEVSTOP/Communicable State Machine(CSM)/addons/API-String-Arugments-Support/_Support/StringAnalyze/check if brackets Matched 2.vi", path "C:/Program Files (x86)/National Instruments/LabVIEW 2017/user.lib/_NEVSTOP/Communicable State Machine(CSM)/addons/API-String-Arugments-Support/_Support/StringAnalyze/check if brackets Matched.vi", path "C:/Program Files (x86)/National Instruments/LabVIEW 2017/user.lib/_NEVSTOP/Communicable State Machine(CSM)/addons/API-String-Arugments-Support/_Support/StringAnalyze/Get content in brackets.vi", path "C:/Program Files (x86)/National Instruments/LabVIEW 2017/user.lib/_NEVSTOP/Communicable State Machine(CSM)/addons/API-String-Arugments-Support/_Support/StringAnalyze/String to 1D Array 2.vi", path "C:/Program Files (x86)/National Instruments/LabVIEW 2017/user.lib/_NEVSTOP/Communicable State Machine(CSM)/addons/API-String-Arugments-Support/_Support/StringAnalyze/Strip brackets with Option.vi", path "C:/Program Files (x86)/National Instruments/LabVIEW 2017/user.lib/_NEVSTOP/Communicable State Machine(CSM)/addons/API-String-Arugments-Support/_Support/StringAnalyze/Strip brackets.vi", path "C:/Program Files (x86)/National Instruments/LabVIEW 2017/user.lib/_NEVSTOP/Communicable State Machine(CSM)/addons/Logger/CSM - Start File Logger.vi", path "C:/Program Files (x86)/National Instruments/LabVIEW 2017/user.lib/_NEVSTOP/Communicable State Machine(CSM)/addons/Logger/CSM File Logger Limit.ctl", path "C:/Program Files (x86)/National Instruments/LabVIEW 2017/user.lib/_NEVSTOP/Communicable State Machine(CSM)/addons/Logger/CSM File Logger.lvlib", path "C:/Program Files (x86)/National Instruments/LabVIEW 2017/user.lib/_NEVSTOP/Communicable State Machine(CSM)/addons/Logger/CSM-Logger-Thread.vi", path "C:/Program Files (x86)/National Instruments/LabVIEW 2017/user.lib/_NEVSTOP/Communicable State Machine(CSM)/addons/Logger/dir.mnu", path "C:/Program Files (x86)/National Instruments/LabVIEW 2017/user.lib/_NEVSTOP/Communicable State Machine(CSM)/addons/Logger/_Support/Append Application Directory If Relative.vi", path "C:/Program Files (x86)/National Instruments/LabVIEW 2017/user.lib/_NEVSTOP/Communicable State Machine(CSM)/addons/Logger/_Support/Convert File Extension (Path)__ogtk.vi", path "C:/Program Files (x86)/National Instruments/LabVIEW 2017/user.lib/_NEVSTOP/Communicable State Machine(CSM)/addons/Logger/_Support/Convert File Extension (String)__ogtk.vi", path "C:/Program Files (x86)/National Instruments/LabVIEW 2017/user.lib/_NEVSTOP/Communicable State Machine(CSM)/addons/Logger/_Support/List Rules as Strings.vi", path "C:/Program Files (x86)/National Instruments/LabVIEW 2017/user.lib/_NEVSTOP/Communicable State Machine(CSM)/addons/Loop-Support/CSM Loop Support.lvlib", path "C:/Program Files (x86)/National Instruments/LabVIEW 2017/user.lib/_NEVSTOP/Communicable State Machine(CSM)/addons/Loop-Support/CSMLS - Add Exit State(s) with Loop Check.vi", path "C:/Program Files (x86)/National Instruments/LabVIEW 2017/user.lib/_NEVSTOP/Communicable State Machine(CSM)/addons/Loop-Support/CSMLS - Append Continuous State.vi", path "C:/Program Files (x86)/National Instruments/LabVIEW 2017/user.lib/_NEVSTOP/Communicable State Machine(CSM)/addons/Loop-Support/CSMLS - Define Loop State(s).vi", path "C:/Program Files (x86)/National Instruments/LabVIEW 2017/user.lib/_NEVSTOP/Communicable State Machine(CSM)/addons/Loop-Support/CSMLS - Remove Loop Tag and previous State(s) to Break.vi", path "C:/Program Files (x86)/National Instruments/LabVIEW 2017/user.lib/_NEVSTOP/Communicable State Machine(CSM)/addons/Loop-Support/CSMLS - Remove Loop Tag to Break.vi", path "C:/Program Files (x86)/National Instruments/LabVIEW 2017/user.lib/_NEVSTOP/Communicable State Machine(CSM)/addons/Loop-Support/dir.mnu", path "C:/Program Files (x86)/National Instruments/LabVIEW 2017/user.lib/_NEVSTOP/Communicable State Machine(CSM)/addons/MassData-Parameter/CSM - Config MassData Parameter Cache Size.vi", path "C:/Program Files (x86)/National Instruments/LabVIEW 2017/user.lib/_NEVSTOP/Communicable State Machine(CSM)/addons/MassData-Parameter/CSM - Convert Argument to MassData.vim", path "C:/Program Files (x86)/National Instruments/LabVIEW 2017/user.lib/_NEVSTOP/Communicable State Machine(CSM)/addons/MassData-Parameter/CSM - Convert MassData to Argument With DataType.vim", path "C:/Program Files (x86)/National Instruments/LabVIEW 2017/user.lib/_NEVSTOP/Communicable State Machine(CSM)/addons/MassData-Parameter/CSM - Convert MassData to Argument.vim", path "C:/Program Files (x86)/National Instruments/LabVIEW 2017/user.lib/_NEVSTOP/Communicable State Machine(CSM)/addons/MassData-Parameter/CSM - MassData Data Type String.vi", path "C:/Program Files (x86)/National Instruments/LabVIEW 2017/user.lib/_NEVSTOP/Communicable State Machine(CSM)/addons/MassData-Parameter/CSM - MassData Parameter Status.vi", path "C:/Program Files (x86)/National Instruments/LabVIEW 2017/user.lib/_NEVSTOP/Communicable State Machine(CSM)/addons/MassData-Parameter/CSM MassData Parameter Support.lvlib", path "C:/Program Files (x86)/National Instruments/LabVIEW 2017/user.lib/_NEVSTOP/Communicable State Machine(CSM)/addons/MassData-Parameter/dir.mnu", path "C:/Program Files (x86)/National Instruments/LabVIEW 2017/user.lib/_NEVSTOP/Communicable State Machine(CSM)/addons/MassData-Parameter/_support/Def-MassDataOper-Status.ctl", path "C:/Program Files (x86)/National Instruments/LabVIEW 2017/user.lib/_NEVSTOP/Communicable State Machine(CSM)/addons/MassData-Parameter/_support/FGV-MassData.vi", path "C:/Program Files (x86)/National Instruments/LabVIEW 2017/user.lib/_NEVSTOP/Communicable State Machine(CSM)/addons/MassData-Parameter/_support/Operation-FGV-MassData.ctl", path "C:/Program Files (x86)/National Instruments/LabVIEW 2017/user.lib/_NEVSTOP/Communicable State Machine(CSM)/addons/MassData-Parameter/Utility/CSM - MassData Update Status Indicator.vi", path "C:/Program Files (x86)/National Instruments/LabVIEW 2017/user.lib/_NEVSTOP/Communicable State Machine(CSM)/addons/MassData-Parameter/Utility/Def-MassData Status Indicator(Horizontal).ctl", path "C:/Program Files (x86)/National Instruments/LabVIEW 2017/user.lib/_NEVSTOP/Communicable State Machine(CSM)/addons/MassData-Parameter/Utility/Def-MassData Status Indicator(Vertical).ctl", path "C:/Program Files (x86)/National Instruments/LabVIEW 2017/user.lib/_NEVSTOP/Communicable State Machine(CSM)/addons/MassData-Parameter/Utility/dir.mnu", path "C:/Program Files (x86)/National Instruments/LabVIEW 2017/user.lib/_NEVSTOP/Communicable State Machine(CSM)/addons/Watchdog/CSM - Start Watchdog to Ensure All Modules Exit.vi", path "C:/Program Files (x86)/National Instruments/LabVIEW 2017/user.lib/_NEVSTOP/Communicable State Machine(CSM)/addons/Watchdog/CSM Watchdog.lvlib", path "C:/Program Files (x86)/National Instruments/LabVIEW 2017/user.lib/_NEVSTOP/Communicable State Machine(CSM)/addons/Watchdog/dir.mnu", path "C:/Program Files (x86)/National Instruments/LabVIEW 2017/user.lib/_NEVSTOP/Communicable State Machine(CSM)/addons/Watchdog/_support/CSM Watchdog Thread.vi", path "C:/Program Files (x86)/National Instruments/LabVIEW 2017/user.lib/_NEVSTOP/Communicable State Machine(CSM)/AdvanceAPI/All Advance APIs.mnu", path "C:/Program Files (x86)/National Instruments/LabVIEW 2017/user.lib/_NEVSTOP/Communicable State Machine(CSM)/AdvanceAPI/Arguments.mnu", path "C:/Program Files (x86)/National Instruments/LabVIEW 2017/user.lib/_NEVSTOP/Communicable State Machine(CSM)/AdvanceAPI/Broadcast Registry.mnu", path "C:/Program Files (x86)/National Instruments/LabVIEW 2017/user.lib/_NEVSTOP/Communicable State Machine(CSM)/AdvanceAPI/Chain Mode.mnu", path "C:/Program Files (x86)/National Instruments/LabVIEW 2017/user.lib/_NEVSTOP/Communicable State Machine(CSM)/AdvanceAPI/CSM - Break Down Multiple States String.vi", path "C:/Program Files (x86)/National Instruments/LabVIEW 2017/user.lib/_NEVSTOP/Communicable State Machine(CSM)/AdvanceAPI/CSM - Broadcast Message Type.ctl", path "C:/Program Files (x86)/National Instruments/LabVIEW 2017/user.lib/_NEVSTOP/Communicable State Machine(CSM)/AdvanceAPI/CSM - Broadcast Status Change.vi", path "C:/Program Files (x86)/National Instruments/LabVIEW 2017/user.lib/_NEVSTOP/Communicable State Machine(CSM)/AdvanceAPI/CSM - Build Exit Messages of CSMs.vi", path "C:/Program Files (x86)/National Instruments/LabVIEW 2017/user.lib/_NEVSTOP/Communicable State Machine(CSM)/AdvanceAPI/CSM - Check If Module Exists.vi", path "C:/Program Files (x86)/National Instruments/LabVIEW 2017/user.lib/_NEVSTOP/Communicable State Machine(CSM)/AdvanceAPI/CSM - Check Mapping Relationship in Broadcast Registry.vi", path "C:/Program Files (x86)/National Instruments/LabVIEW 2017/user.lib/_NEVSTOP/Communicable State Machine(CSM)/AdvanceAPI/CSM - Compact Multiple States.vi", path "C:/Program Files (x86)/National Instruments/LabVIEW 2017/user.lib/_NEVSTOP/Communicable State Machine(CSM)/AdvanceAPI/CSM - Convert Argument to Error.vi", path "C:/Program Files (x86)/National Instruments/LabVIEW 2017/user.lib/_NEVSTOP/Communicable State Machine(CSM)/AdvanceAPI/CSM - Convert Data to HexStr.vi", path "C:/Program Files (x86)/National Instruments/LabVIEW 2017/user.lib/_NEVSTOP/Communicable State Machine(CSM)/AdvanceAPI/CSM - Convert Error to Argument.vi", path "C:/Program Files (x86)/National Instruments/LabVIEW 2017/user.lib/_NEVSTOP/Communicable State Machine(CSM)/AdvanceAPI/CSM - Convert Filter Rules.vi", path "C:/Program Files (x86)/National Instruments/LabVIEW 2017/user.lib/_NEVSTOP/Communicable State Machine(CSM)/AdvanceAPI/CSM - Convert HexStr to Data.vi", path "C:/Program Files (x86)/National Instruments/LabVIEW 2017/user.lib/_NEVSTOP/Communicable State Machine(CSM)/AdvanceAPI/CSM - Destroy Global Log Event.vi", path "C:/Program Files (x86)/National Instruments/LabVIEW 2017/user.lib/_NEVSTOP/Communicable State Machine(CSM)/AdvanceAPI/CSM - Destroy Status Change Event.vi", path "C:/Program Files (x86)/National Instruments/LabVIEW 2017/user.lib/_NEVSTOP/Communicable State Machine(CSM)/AdvanceAPI/CSM - Filter Duplicate Messages By Name.vi", path "C:/Program Files (x86)/National Instruments/LabVIEW 2017/user.lib/_NEVSTOP/Communicable State Machine(CSM)/AdvanceAPI/CSM - Filter Global Log.vi", path "C:/Program Files (x86)/National Instruments/LabVIEW 2017/user.lib/_NEVSTOP/Communicable State Machine(CSM)/AdvanceAPI/CSM - Filter Messages to Non-Existing Modules.vi", path "C:/Program Files (x86)/National Instruments/LabVIEW 2017/user.lib/_NEVSTOP/Communicable State Machine(CSM)/AdvanceAPI/CSM - Forward States to CSM.vi", path "C:/Program Files (x86)/National Instruments/LabVIEW 2017/user.lib/_NEVSTOP/Communicable State Machine(CSM)/AdvanceAPI/CSM - Forward UI Operations to CSM.vi", path "C:/Program Files (x86)/National Instruments/LabVIEW 2017/user.lib/_NEVSTOP/Communicable State Machine(CSM)/AdvanceAPI/CSM - Generate User Global Log.vi", path "C:/Program Files (x86)/National Instruments/LabVIEW 2017/user.lib/_NEVSTOP/Communicable State Machine(CSM)/AdvanceAPI/CSM - Get New State Notifier Event.vi", path "C:/Program Files (x86)/National Instruments/LabVIEW 2017/user.lib/_NEVSTOP/Communicable State Machine(CSM)/AdvanceAPI/CSM - Global Log Error Handler.vi", path "C:/Program Files (x86)/National Instruments/LabVIEW 2017/user.lib/_NEVSTOP/Communicable State Machine(CSM)/AdvanceAPI/CSM - Global Log Event.vi", path "C:/Program Files (x86)/National Instruments/LabVIEW 2017/user.lib/_NEVSTOP/Communicable State Machine(CSM)/AdvanceAPI/CSM - Internal State Debug Log History.vi", path "C:/Program Files (x86)/National Instruments/LabVIEW 2017/user.lib/_NEVSTOP/Communicable State Machine(CSM)/AdvanceAPI/CSM - Keywords.vi", path "C:/Program Files (x86)/National Instruments/LabVIEW 2017/user.lib/_NEVSTOP/Communicable State Machine(CSM)/AdvanceAPI/CSM - List Log Filter Rules As Strings.vi", path "C:/Program Files (x86)/National Instruments/LabVIEW 2017/user.lib/_NEVSTOP/Communicable State Machine(CSM)/AdvanceAPI/CSM - List Mapping Relationships in Broadcast Registry.vi", path "C:/Program Files (x86)/National Instruments/LabVIEW 2017/user.lib/_NEVSTOP/Communicable State Machine(CSM)/AdvanceAPI/CSM - List Modules.vi", path "C:/Program Files (x86)/National Instruments/LabVIEW 2017/user.lib/_NEVSTOP/Communicable State Machine(CSM)/AdvanceAPI/CSM - List Rules in Broadcast Registry.vi", path "C:/Program Files (x86)/National Instruments/LabVIEW 2017/user.lib/_NEVSTOP/Communicable State Machine(CSM)/AdvanceAPI/CSM - List Status in Broadcast Registry.vi", path "C:/Program Files (x86)/National Instruments/LabVIEW 2017/user.lib/_NEVSTOP/Communicable State Machine(CSM)/AdvanceAPI/CSM - Make String Arguments Safe.vi", path "C:/Program Files (x86)/National Instruments/LabVIEW 2017/user.lib/_NEVSTOP/Communicable State Machine(CSM)/AdvanceAPI/CSM - Mark As Chain Module.vi", path "C:/Program Files (x86)/National Instruments/LabVIEW 2017/user.lib/_NEVSTOP/Communicable State Machine(CSM)/AdvanceAPI/CSM - Mark As Worker Module.vi", path "C:/Program Files (x86)/National Instruments/LabVIEW 2017/user.lib/_NEVSTOP/Communicable State Machine(CSM)/AdvanceAPI/CSM - Message Type.ctl", path "C:/Program Files (x86)/National Instruments/LabVIEW 2017/user.lib/_NEVSTOP/Communicable State Machine(CSM)/AdvanceAPI/CSM - Module Exit Event.vi", path "C:/Program Files (x86)/National Instruments/LabVIEW 2017/user.lib/_NEVSTOP/Communicable State Machine(CSM)/AdvanceAPI/CSM - Module Status.vi", path "C:/Program Files (x86)/National Instruments/LabVIEW 2017/user.lib/_NEVSTOP/Communicable State Machine(CSM)/AdvanceAPI/CSM - Module Turns Invalid.vi", path "C:/Program Files (x86)/National Instruments/LabVIEW 2017/user.lib/_NEVSTOP/Communicable State Machine(CSM)/AdvanceAPI/CSM - Module VI Reference.vi", path "C:/Program Files (x86)/National Instruments/LabVIEW 2017/user.lib/_NEVSTOP/Communicable State Machine(CSM)/AdvanceAPI/CSM - Post Message.vi", path "C:/Program Files (x86)/National Instruments/LabVIEW 2017/user.lib/_NEVSTOP/Communicable State Machine(CSM)/AdvanceAPI/CSM - Register Status Change.vi", path "C:/Program Files (x86)/National Instruments/LabVIEW 2017/user.lib/_NEVSTOP/Communicable State Machine(CSM)/AdvanceAPI/CSM - Remove Duplicated Following Messages.vi", path "C:/Program Files (x86)/National Instruments/LabVIEW 2017/user.lib/_NEVSTOP/Communicable State Machine(CSM)/AdvanceAPI/CSM - Remove Module in Broadcast Registry.vi", path "C:/Program Files (x86)/National Instruments/LabVIEW 2017/user.lib/_NEVSTOP/Communicable State Machine(CSM)/AdvanceAPI/CSM - Replace Substitution Marks in Messages.vi", path "C:/Program Files (x86)/National Instruments/LabVIEW 2017/user.lib/_NEVSTOP/Communicable State Machine(CSM)/AdvanceAPI/CSM - Request CSM to Broadcast Status Change.vi", path "C:/Program Files (x86)/National Instruments/LabVIEW 2017/user.lib/_NEVSTOP/Communicable State Machine(CSM)/AdvanceAPI/CSM - Request CSM to Post Message.vi", path "C:/Program Files (x86)/National Instruments/LabVIEW 2017/user.lib/_NEVSTOP/Communicable State Machine(CSM)/AdvanceAPI/CSM - Revert Arguments-Safe String.vi", path "C:/Program Files (x86)/National Instruments/LabVIEW 2017/user.lib/_NEVSTOP/Communicable State Machine(CSM)/AdvanceAPI/CSM - Run Script.vi", path "C:/Program Files (x86)/National Instruments/LabVIEW 2017/user.lib/_NEVSTOP/Communicable State Machine(CSM)/AdvanceAPI/CSM - Send Message and Wait for Reply.vi", path "C:/Program Files (x86)/National Instruments/LabVIEW 2017/user.lib/_NEVSTOP/Communicable State Machine(CSM)/AdvanceAPI/CSM - Set Log Filter Rules.vi", path "C:/Program Files (x86)/National Instruments/LabVIEW 2017/user.lib/_NEVSTOP/Communicable State Machine(CSM)/AdvanceAPI/CSM - Status Change Event.vi", path "C:/Program Files (x86)/National Instruments/LabVIEW 2017/user.lib/_NEVSTOP/Communicable State Machine(CSM)/AdvanceAPI/CSM - Unregister Status Change.vi", path "C:/Program Files (x86)/National Instruments/LabVIEW 2017/user.lib/_NEVSTOP/Communicable State Machine(CSM)/AdvanceAPI/CSM - Wait and Post Message.vi", path "C:/Program Files (x86)/National Instruments/LabVIEW 2017/user.lib/_NEVSTOP/Communicable State Machine(CSM)/AdvanceAPI/CSM - Wait and Send Message for Reply.vi", path "C:/Program Files (x86)/National Instruments/LabVIEW 2017/user.lib/_NEVSTOP/Communicable State Machine(CSM)/AdvanceAPI/CSM - Wait for All Modules to be Alive.vi", path "C:/Program Files (x86)/National Instruments/LabVIEW 2017/user.lib/_NEVSTOP/Communicable State Machine(CSM)/AdvanceAPI/CSM - Wait for All Modules to Exit.vi", path "C:/Program Files (x86)/National Instruments/LabVIEW 2017/user.lib/_NEVSTOP/Communicable State Machine(CSM)/AdvanceAPI/CSM - Wait for Module to Be Alive.vi", path "C:/Program Files (x86)/National Instruments/LabVIEW 2017/user.lib/_NEVSTOP/Communicable State Machine(CSM)/AdvanceAPI/dir.mnu", path "C:/Program Files (x86)/National Instruments/LabVIEW 2017/user.lib/_NEVSTOP/Communicable State Machine(CSM)/AdvanceAPI/Global Log Event.mnu", path "C:/Program Files (x86)/National Instruments/LabVIEW 2017/user.lib/_NEVSTOP/Communicable State Machine(CSM)/AdvanceAPI/HelperVIs.mnu", path "C:/Program Files (x86)/National Instruments/LabVIEW 2017/user.lib/_NEVSTOP/Communicable State Machine(CSM)/AdvanceAPI/Non-CSM Caller Support.mnu", path "C:/Program Files (x86)/National Instruments/LabVIEW 2017/user.lib/_NEVSTOP/Communicable State Machine(CSM)/AdvanceAPI/Side Loop Support.mnu", path "C:/Program Files (x86)/National Instruments/LabVIEW 2017/user.lib/_NEVSTOP/Communicable State Machine(CSM)/AdvanceAPI/Worker Mode.mnu", path "C:/Program Files (x86)/National Instruments/LabVIEW 2017/user.lib/_NEVSTOP/Communicable State Machine(CSM)/More Templates/More Templates.mnu", path "C:/Program Files (x86)/National Instruments/LabVIEW 2017/user.lib/_NEVSTOP/Communicable State Machine(CSM)/Utility/Build Error Cluster.vi", path "C:/Program Files (x86)/National Instruments/LabVIEW 2017/user.lib/_NEVSTOP/Communicable State Machine(CSM)/Utility/Build Internal State String.vi", path "C:/Program Files (x86)/National Instruments/LabVIEW 2017/user.lib/_NEVSTOP/Communicable State Machine(CSM)/Utility/Check Timeout.vi", path "C:/Program Files (x86)/National Instruments/LabVIEW 2017/user.lib/_NEVSTOP/Communicable State Machine(CSM)/Utility/CSM Data Type String to Enum.vi", path "C:/Program Files (x86)/National Instruments/LabVIEW 2017/user.lib/_NEVSTOP/Communicable State Machine(CSM)/Utility/CSM Data Type String.vi", path "C:/Program Files (x86)/National Instruments/LabVIEW 2017/user.lib/_NEVSTOP/Communicable State Machine(CSM)/Utility/dir.mnu", path "C:/Program Files (x86)/National Instruments/LabVIEW 2017/user.lib/_NEVSTOP/Communicable State Machine(CSM)/Utility/Global Log History Cacher.vi", path "C:/Program Files (x86)/National Instruments/LabVIEW 2017/user.lib/_NEVSTOP/Communicable State Machine(CSM)/Utility/Global Log To String.vi", path "C:/Program Files (x86)/National Instruments/LabVIEW 2017/user.lib/_NEVSTOP/Communicable State Machine(CSM)/Utility/Match Asterisk Pattern.vi", path "C:/Program Files (x86)/National Instruments/LabVIEW 2017/user.lib/_NEVSTOP/Communicable State Machine(CSM)/Utility/Periodic String Filter Info.ctl", path "C:/Program Files (x86)/National Instruments/LabVIEW 2017/user.lib/_NEVSTOP/Communicable State Machine(CSM)/Utility/Periodic String Filter State.ctl", path "C:/Program Files (x86)/National Instruments/LabVIEW 2017/user.lib/_NEVSTOP/Communicable State Machine(CSM)/Utility/Periodic String Filter.vi", path "C:/Program Files (x86)/National Instruments/LabVIEW 2017/user.lib/_NEVSTOP/Communicable State Machine(CSM)/Utility/Random Change Flag.vi", path "C:/Program Files (x86)/National Instruments/LabVIEW 2017/user.lib/_NEVSTOP/Communicable State Machine(CSM)/Utility/Replace Tag with Array.vi", path "C:/Program Files (x86)/National Instruments/LabVIEW 2017/user.lib/_NEVSTOP/Communicable State Machine(CSM)/Utility/String History Cacher.vi", path "C:/Program Files (x86)/National Instruments/LabVIEW 2017/user.lib/_NEVSTOP/Communicable State Machine(CSM)/Utility/Timeout Selector.vi", path "C:/Program Files (x86)/National Instruments/LabVIEW 2017/user.lib/_NEVSTOP/Communicable State Machine(CSM)/Utility/Trim Both Whitespace.vi", path "C:/Program Files (x86)/National Instruments/LabVIEW 2017/user.lib/_NEVSTOP/Communicable State Machine(CSM)/Utility/uuid.vi", path "C:/Program Files (x86)/National Instruments/LabVIEW 2017/user.lib/_NEVSTOP/Communicable State Machine(CSM)/Utility/_openG/1D Array to String_csm.vi", path "C:/Program Files (x86)/National Instruments/LabVIEW 2017/user.lib/_NEVSTOP/Communicable State Machine(CSM)/Utility/_openG/Array of VData to VCluster_csm.vi", path "C:/Program Files (x86)/National Instruments/LabVIEW 2017/user.lib/_NEVSTOP/Communicable State Machine(CSM)/Utility/_openG/End of Line Constant (bug fix)_csm.vi", path "C:/Program Files (x86)/National Instruments/LabVIEW 2017/user.lib/_NEVSTOP/Communicable State Machine(CSM)/Utility/_openG/Get Data Name_csm.vi", path "C:/Program Files (x86)/National Instruments/LabVIEW 2017/user.lib/_NEVSTOP/Communicable State Machine(CSM)/Utility/_openG/Get Header from TD_csm.vi", path "C:/Program Files (x86)/National Instruments/LabVIEW 2017/user.lib/_NEVSTOP/Communicable State Machine(CSM)/Utility/_openG/Get Last PString_csm.vi", path "C:/Program Files (x86)/National Instruments/LabVIEW 2017/user.lib/_NEVSTOP/Communicable State Machine(CSM)/Utility/_openG/Get PString_csm.vi", path "C:/Program Files (x86)/National Instruments/LabVIEW 2017/user.lib/_NEVSTOP/Communicable State Machine(CSM)/Utility/_openG/Get Strings from Enum_csm.vi", path "C:/Program Files (x86)/National Instruments/LabVIEW 2017/user.lib/_NEVSTOP/Communicable State Machine(CSM)/Utility/_openG/Set Data Name_csm.vi", path "C:/Program Files (x86)/National Instruments/LabVIEW 2017/user.lib/_NEVSTOP/Communicable State Machine(CSM)/Utility/_openG/Set Enum String Value_csm.vi", path "C:/Program Files (x86)/National Instruments/LabVIEW 2017/user.lib/_NEVSTOP/Communicable State Machine(CSM)/Utility/_openG/String to 1D Array_csm.vi", path "C:/Program Files (x86)/National Instruments/LabVIEW 2017/user.lib/_NEVSTOP/Communicable State Machine(CSM)/Utility/_support/CSM Data Type String to Enum(RefnumEnum).vi", path "C:/Program Files (x86)/National Instruments/LabVIEW 2017/user.lib/_NEVSTOP/Communicable State Machine(CSM)/Utility/_support/CSM Data Type String to Enum(String).vi", path "C:/Program Files (x86)/National Instruments/LabVIEW 2017/user.lib/_NEVSTOP/Communicable State Machine(CSM)/Utility/_support/CSM Data Type String to Enum(TypeEnum).vi"]
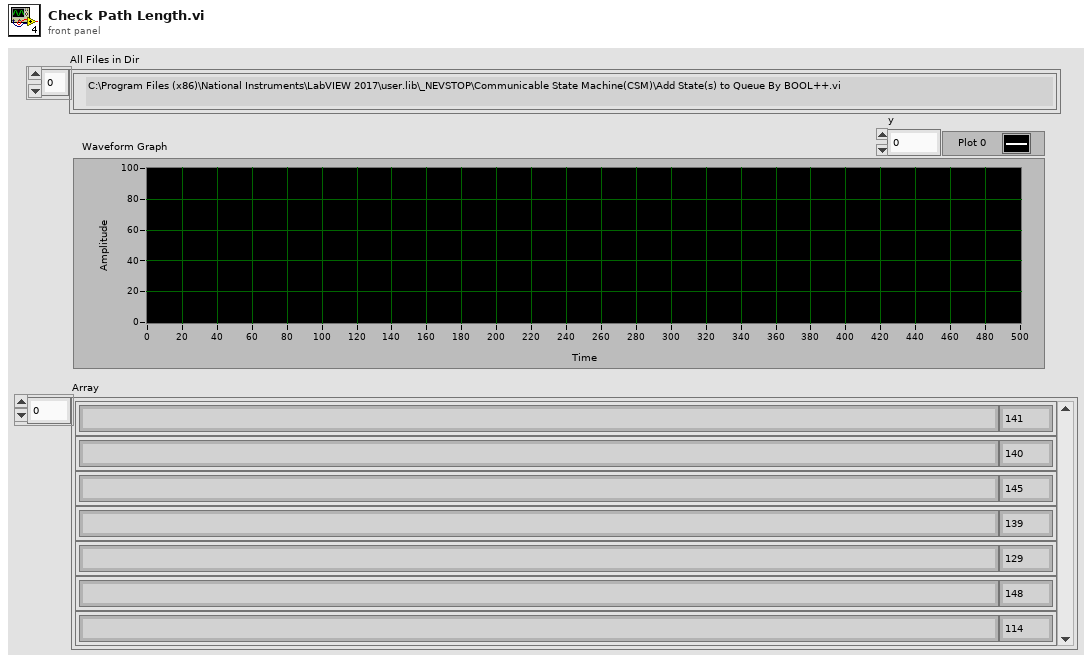
[diagram p1: front panel]
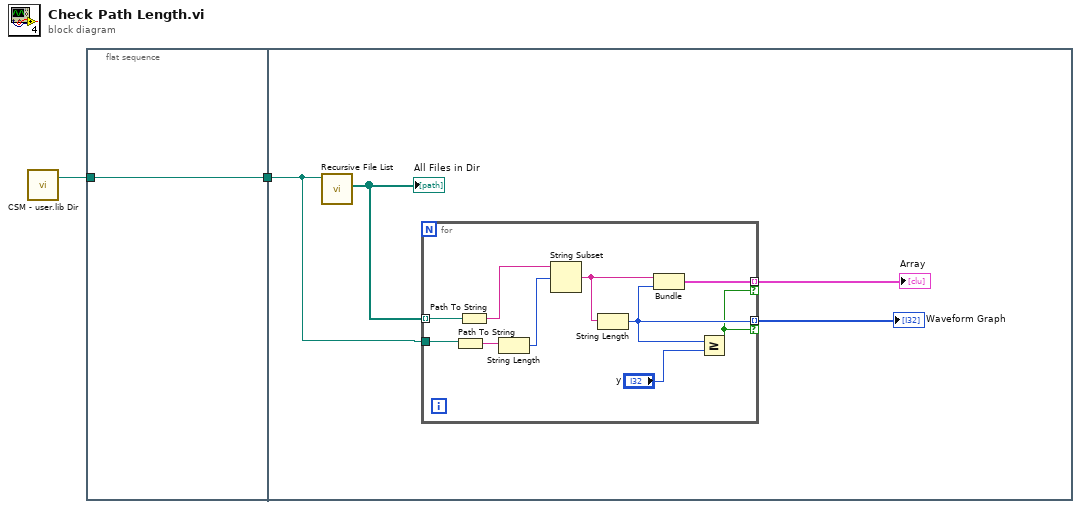
[diagram p0: block diagram]
diagram:
  n1 = call "CSM - user.lib Dir.vi"() -> ("csm_user.lib_dir"=w2:path)  [unwired: 2 in, 1 out]
  n2 = flat-sequence {
    tunnel: w2 -> [w3]
    tunnel: [w3] -> w1
    tunnel: w1 -> [w4]
    frame #0 {
    }
    frame #1 {
      n3 = call <vilib>:"Recursive File List.vi"("Folder Path"=w4) -> ("All Files in Dir"=w7:path[])  [unwired: 6 in, 4 out]
      "All Files in Dir" <- w7
      n4 = for {
        tunnel: w7 -> [w17] mode=indexing
        tunnel: [w15] -> w6 mode=indexing if=w13
        tunnel: [w16] -> w5 mode=indexing if=w13
        tunnel: w4 -> [w12]
        n5 = Path To String(path=w12) -> (string=w10:string)
        n6 = Path To String(path=w17) -> (string=w11:string)
        n7 = String Length(string=w10) -> (length=w9:i32)
        n8 = String Subset(string=w11, offset (0)=w9) -> (substring=w8:string)  [unwired: 1 in]
        n9 = String Length(string=w8) -> (length=w15:i32)
        n10 = Bundle(w8, w15) -> (w16:cluster{string, i32})  [unwired: 1 in]
        n11 = Greater Or Equal?(x=w15, y="y") -> (x >= y?=w13:bool)
      }
      "Waveform Graph" <- w6
      "Array" <- w5
    }
  }
